vi "main_001.vi"() -> ()   [LabVIEW 2016]
uses:
  ISEGNHQxxu/iseg NHQ VISA Control.ctl
  <vilib>/Analysis/1siggen.llb/Ramp Pattern by Samples.vi
  <vilib>/Utility/file.llb/Read From Spreadsheet File (DBL).vi
  <vilib>/Utility/file.llb/Write Delimited Spreadsheet (string).vi
  <vilib>/Utility/file.llb/Write Delimited Spreadsheet (DBL).vi
  <vilib>/Platform/browser.llb/Open URL in Default Browser (path).vi
  <vilib>/Analysis/NI_AALBase.lvlib
  Newport ESP301/Newport ESP301.lvlib
panel:
  out "noise-o-meter":dbl=nan format="%.1g"
  in  "array size":i32
  out "Waveform Chart":dbl(graph)=159723533.31
  in  "open base path":bool
  in  "Path":path=path "Y:/Ediff/data/2017/01/170106"
  in  "stop":bool
  out "Slide":dbl(slide)=0.99 scale=0.0..1.0
  in  "Tab Control":T1(tab)
  out "esp_pos_fs":dbl caption="[fs]" format="%.6g"
  in  "snap":bool
  in  "dark":bool
  in  "savebin":bool
  in  "savepng":bool
  in  "count?":bool
  in  "dark?":bool
  in  "threshold":i32=110
  in  "t_exp":dbl=0.1 caption="Exposure time [s]"
  in  "dark_load":bool
  in  "frames":i32=100
  in  "avg[t] acc[f]":bool=TRUE
  out "Actual Voltage":dbl[unit]=-0.6 format="%.2f"
  in  "volt_set":bool
  in  "Nominal Voltage":sgl=50.0 max=4000 format="%.2f"
  out "[mm]":dbl format="%.6g"
  in  "esp_rel+":bool
  in  "esp_rel-":bool
  in  "esp_abs_go":bool
  in  "esp_rel_delta":dbl=0.1 caption="delta [mm]" min=0.0
  in  "esp_abs_time":dbl caption="[fs]"
  in  "esp_set_t0":bool
  out "t0 @":dbl format="%.6g"
  in  "esp_abs_dest":dbl caption="[mm]"
  in  "Value in":dbl=2.0 caption="binning"
  in  "delayscan_go":bool
  in  "waypoints":string[][](table)=[["-100000", "5000"], ["50000", ""], ["", ""]]
  in  "delayscan_header":string="DelayScan01" caption="header"
  in  "iterations":i32
  out "XY Graph":cluster{"Array":dbl[], dbl[]}(graph)
  in  "delayscan_stop":bool
  out "Slide 2":dbl(slide)=0.999 scale=0.0..1.0
  in  "meas_stop_volt":bool
  in  "meas_start_volt":bool
  in  "head":string="PowerVoltScan1"
  in  "volt_start":dbl format="%0.2f"
  in  "volt_end":dbl=1.0 format="%0.2f"
  in  "volt_samples":i32=128
  in  "move2com":bool
  in  "meas_start_XY":bool
  in  "showcom":bool
  in  "VISA ISEG":refnum<visa-resource-name>="COM6"
  in  "Channel (A)":enum16{"A", "B"}(ring)=enum."B"
  out "error out":errorcluster
  in  "volt_timeout":u32=6000
  in  "volt_threshold":sgl=2.0 max=4000 format="%.2f"
  in  "esp_axis":i32=2 caption="ESP Axis" min=1 max=3
  in  "esp_visa":refnum<visa-resource-name>="COM1" caption="ESP VISA"
  out "esp301":errorcluster={"status"=TRUE, "code"=-1073807346, "source"="VISA Open in Newport ESP301.lvlib:Initialize.vi->main 0.9.vi"}
  out "captured":dbl[][](graph)
  out "live":dbl[][](graph)
  in  "close":bool
  # "%"
  # "camera"
  # "voltage supply"
  # "delay stage"
  # "absolute"
  # "Axis2"
  # "Axis1"
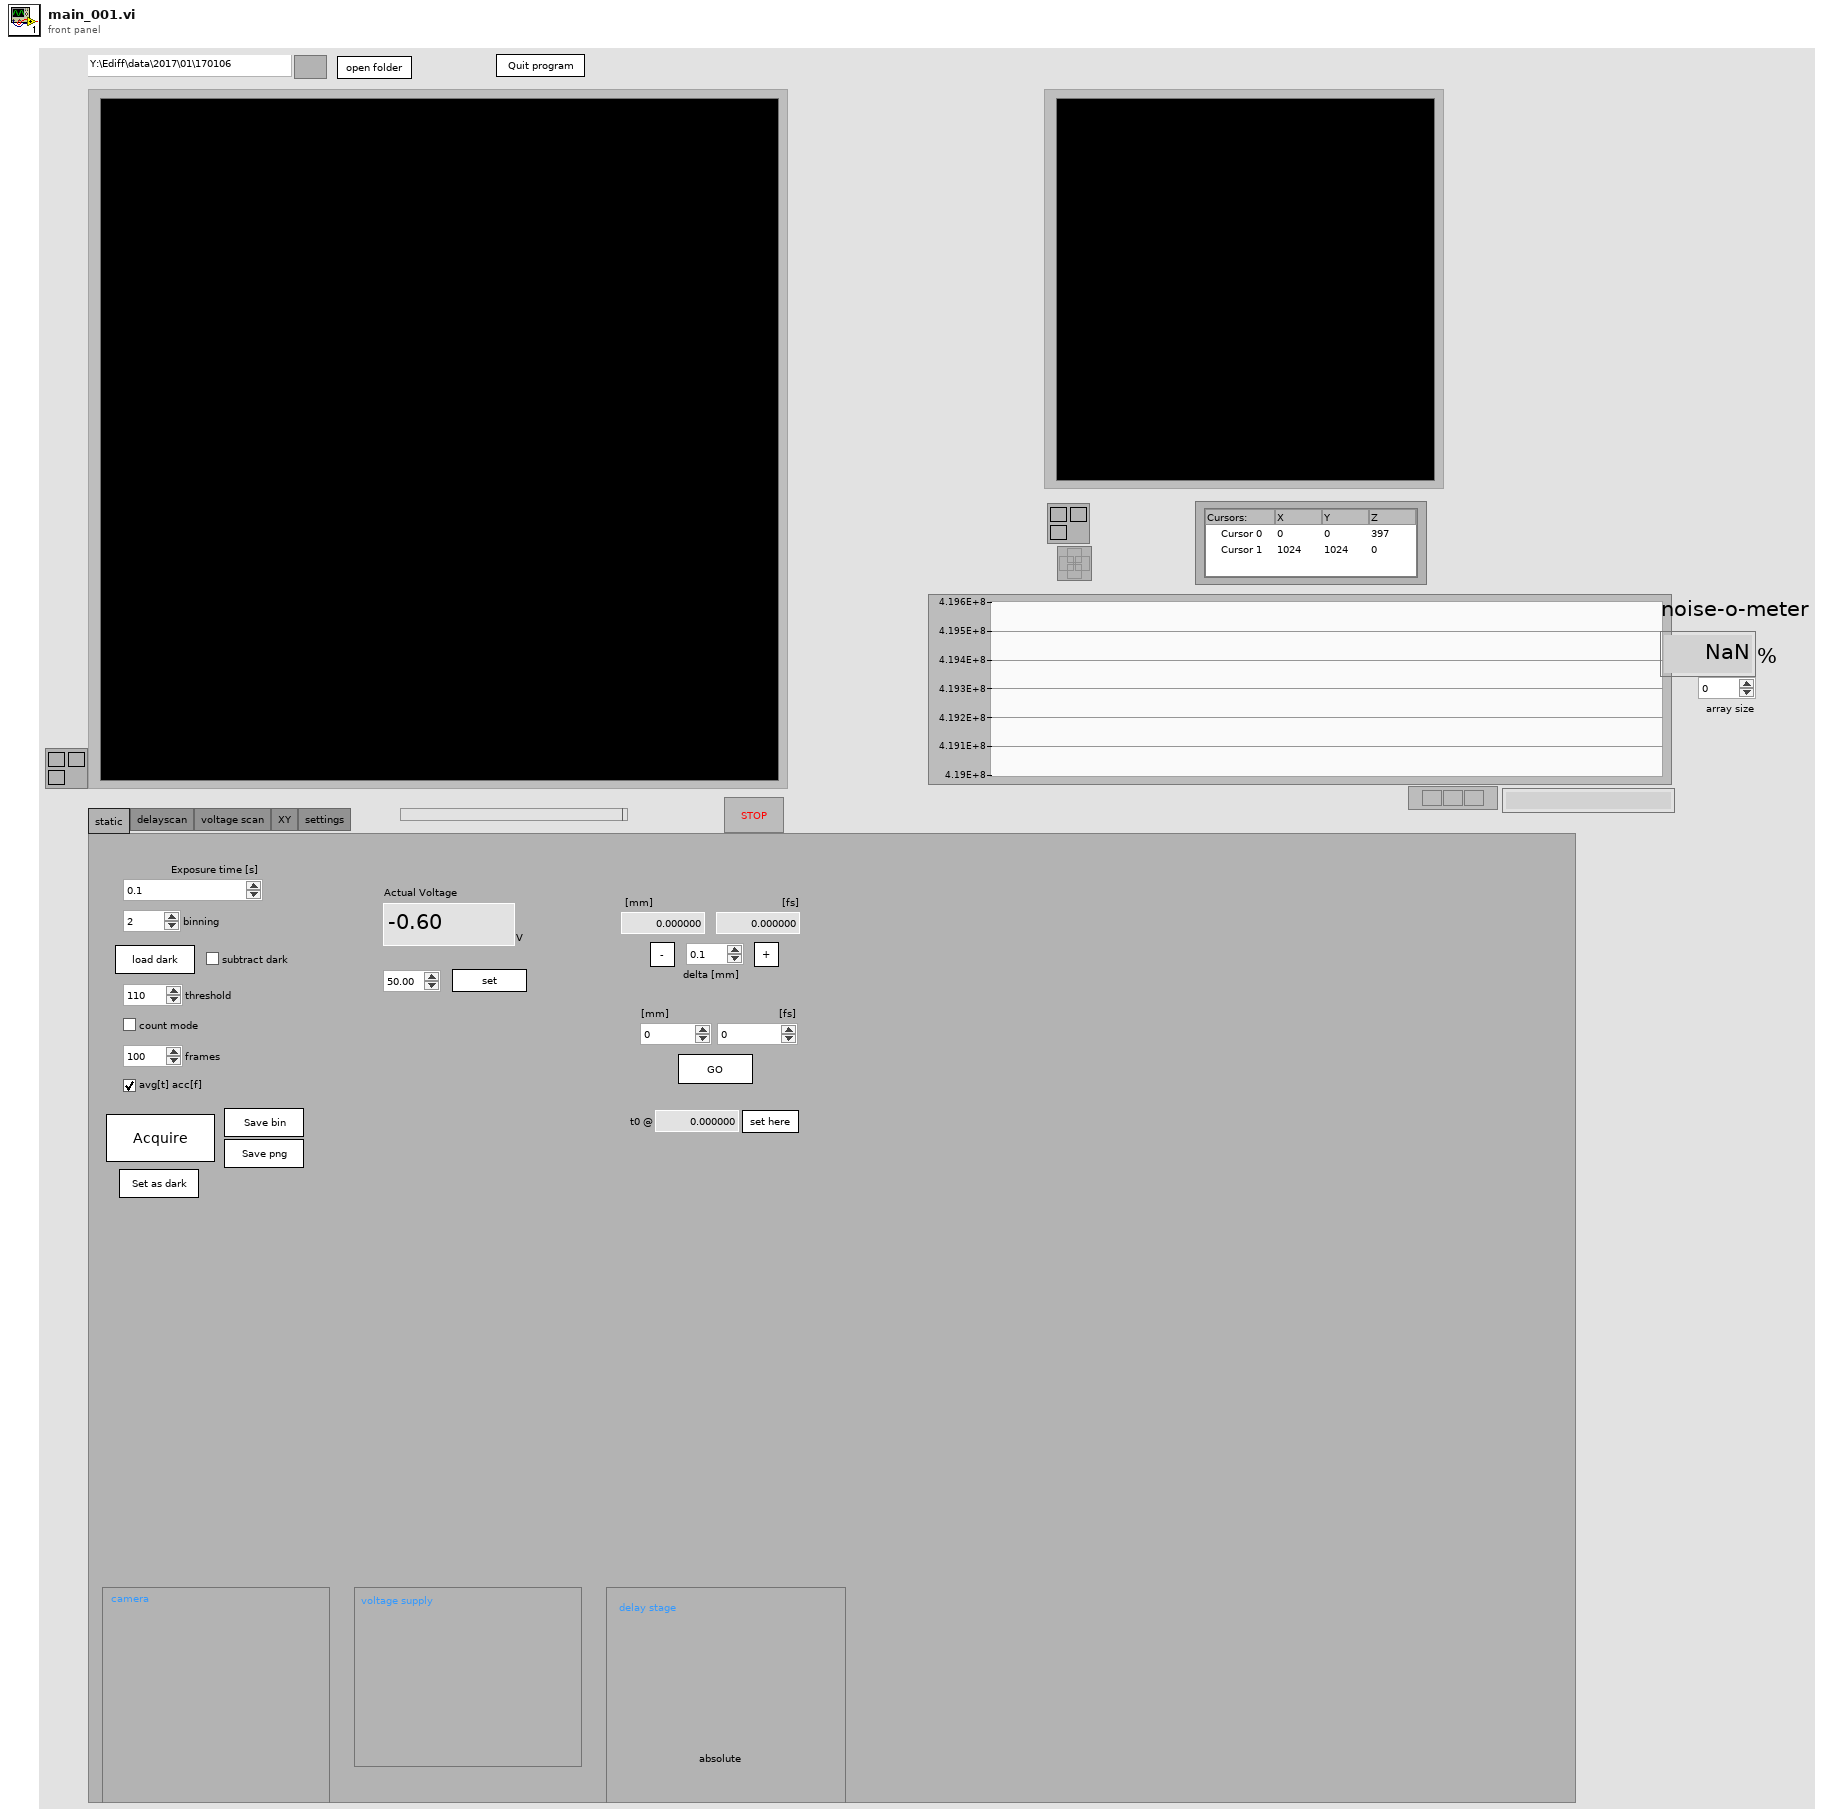
[diagram p1: front panel]
types:
  T1 = enum32{"static", "delayscan", "voltage scan", "XY", "settings"}
  T2 = typedef "Image Type" = u32
  T3 = typedef "IMAQ Image.ctl" = refnum<image>
  T4 = cluster{"height":u32, "width":u32, "datatype":u32}
  T5 = typedef "iseg NHQ VISA Control.ctl" = cluster{"VISA Resource Name":refnum<visa-resource-name>, "FP Notation":bool, "Maximum Voltage":u32, "Maximum Current":u32}
  T6 = cluster{"Axis1 moving":bool, "Axis2 moving":bool, "Axis3 moving":bool, "Axis4 moving":bool, "Motor Power of at least one axis":bool, "Reserved":bool, "Reserved":bool, "Reserved":bool, "Axis5 moving 2":bool, "Axis6 moving 2":bool, "Reserved":bool, "Reserved":bool, "Motor Power of at least one axis":bool, "Reserved":bool, "Reserved":bool, "Reserved":bool}
  T7 = typedef "LVCursorListTypeDef.ctl" = cluster{"Name":string, "Color":u32, "Style":u8, "Point Style":u8, "Name Visible":bool, "Allow Drag":bool, "Cursor Mode":u32, "Plot":i32, "Index":i32, "Position":cluster{"X":dbl, "Y":dbl}, "X Scale":u32, "Y Scale":u32, "Watch Plots":i32[], "Watch All Plots":bool, "Plot Area":i32, "Label Offset":cluster{"X":dbl, "Y":dbl}}[]
  T8 = cluster{"Name":string, "Color":u32, "Style":u8, "Point Style":u8, "Name Visible":bool, "Allow Drag":bool, "Cursor Mode":u32, "Plot":i32, "Index":i32, "Position":cluster{"X":dbl, "Y":dbl}, "X Scale":u32, "Y Scale":u32, "Watch Plots":i32[], "Watch All Plots":bool, "Plot Area":i32, "Label Offset":cluster{"X":dbl, "Y":dbl}}
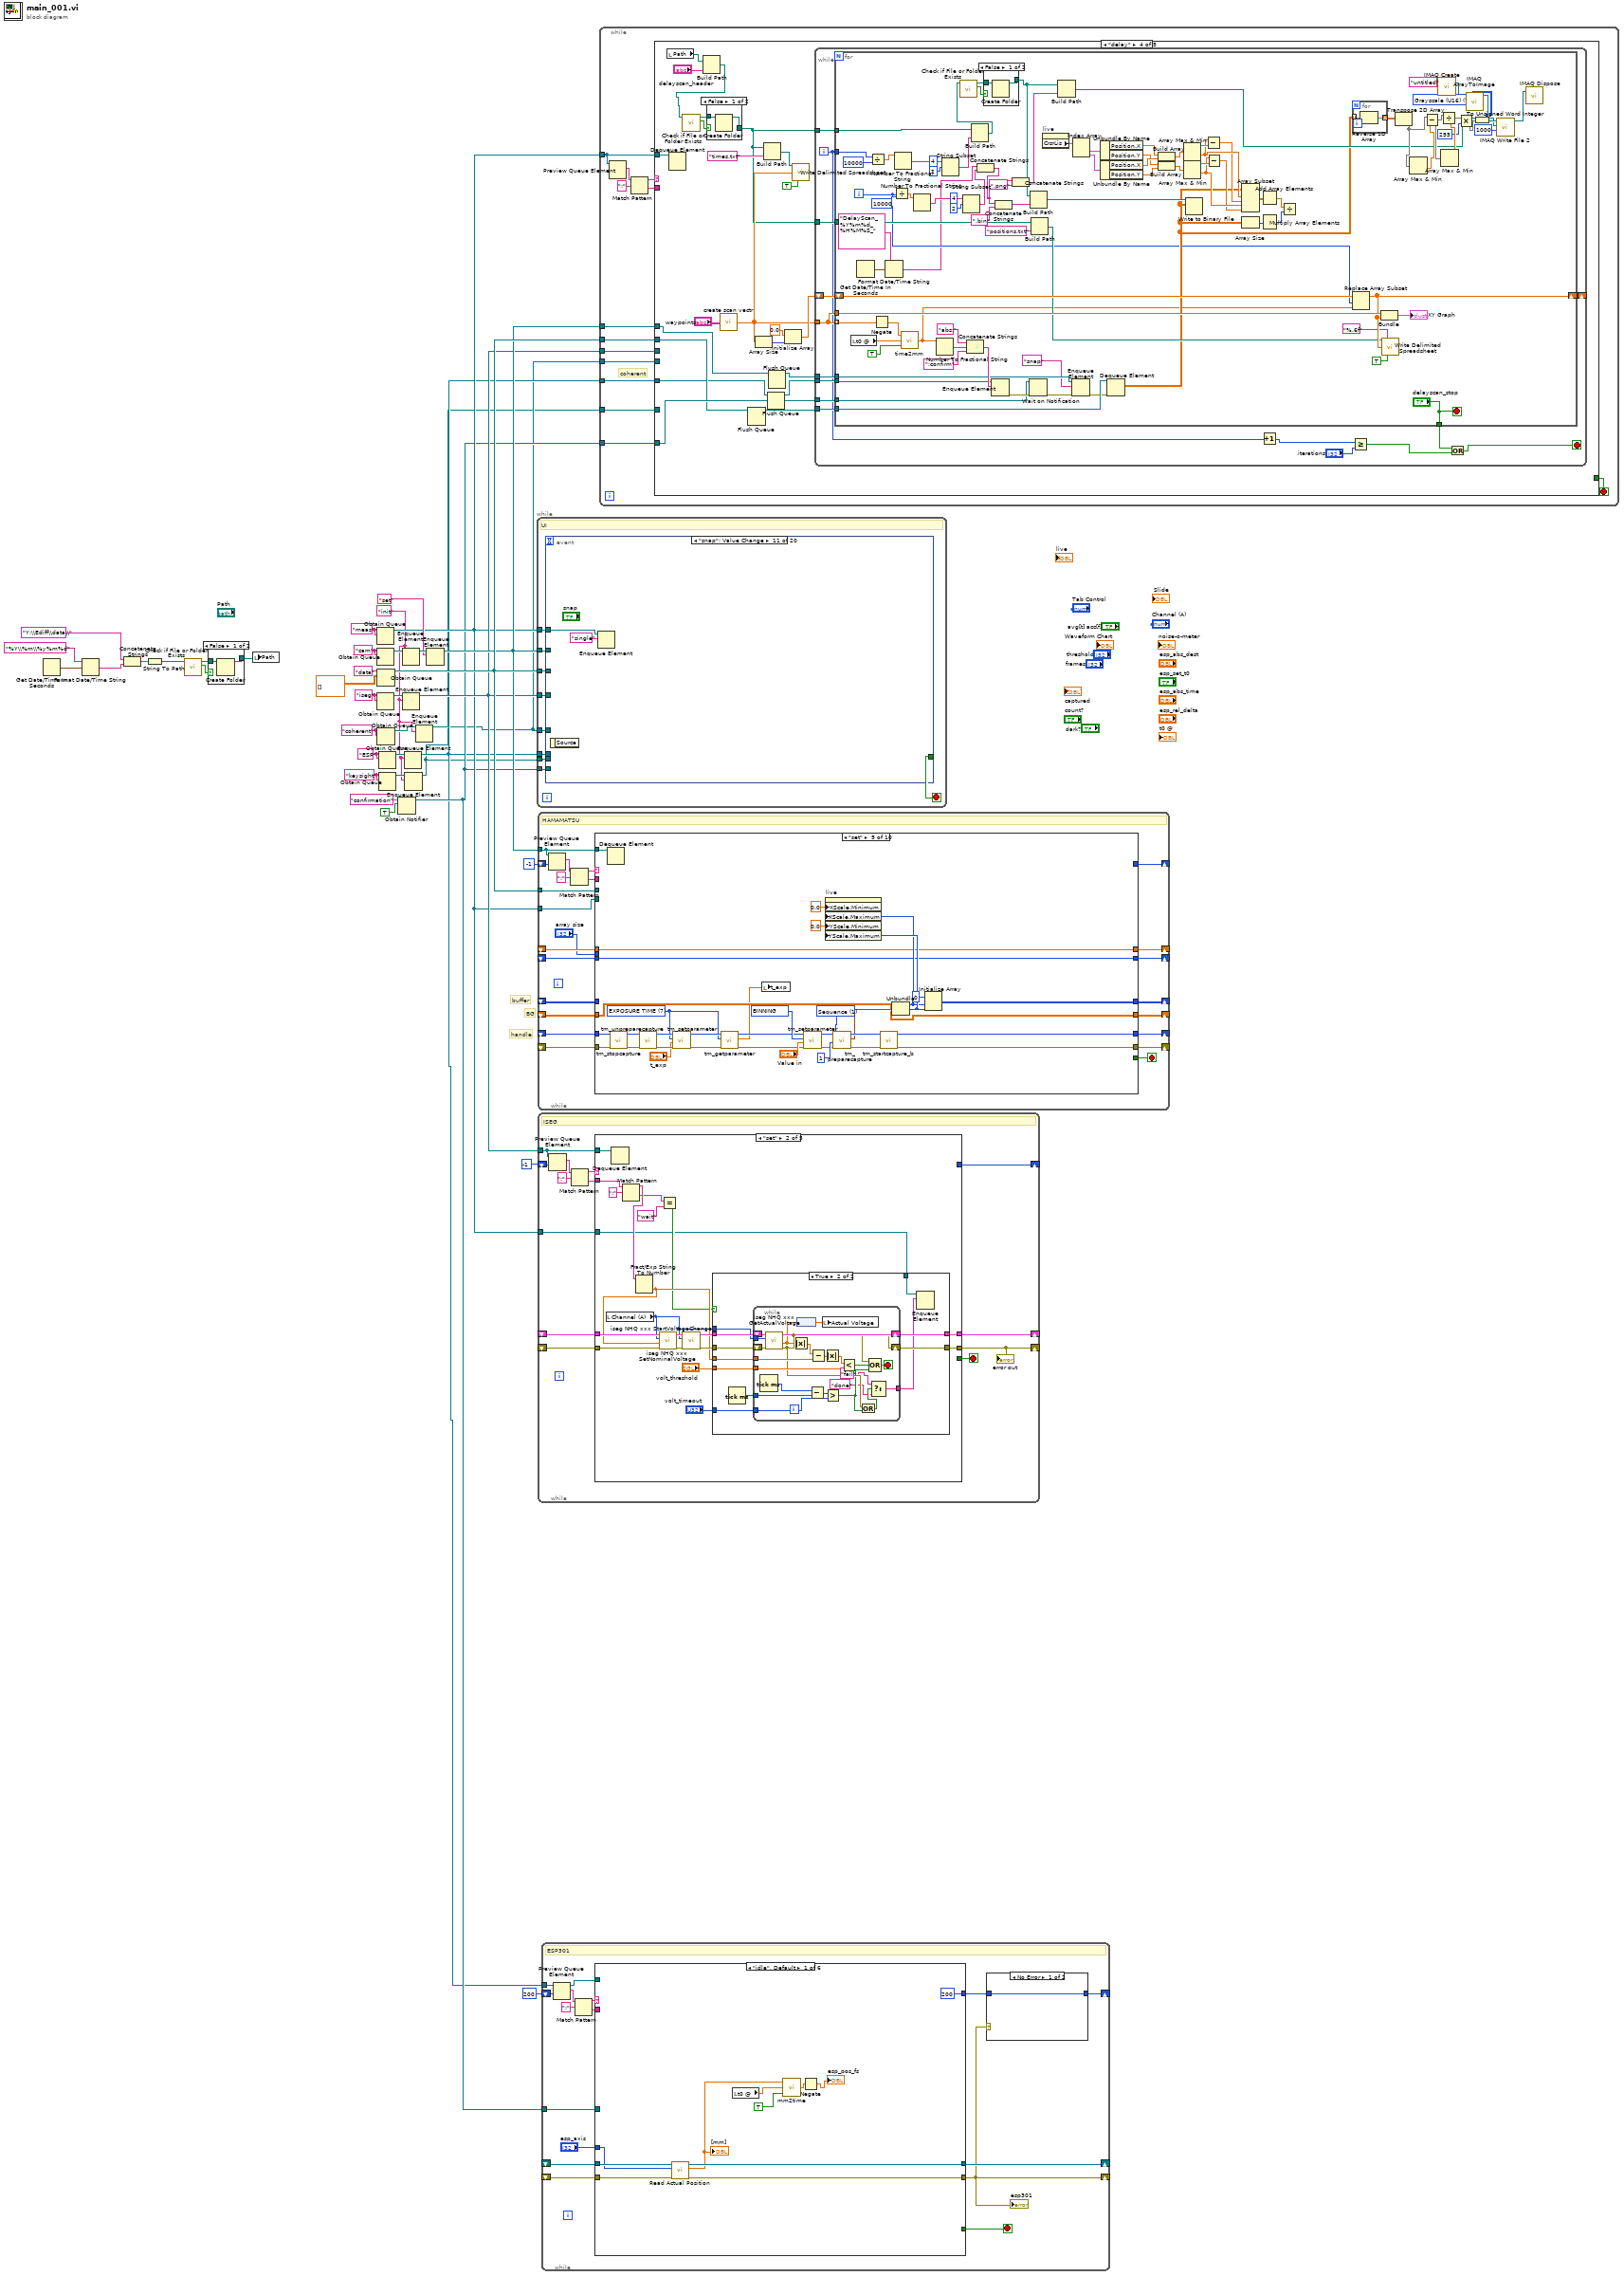
[diagram p0: block diagram]
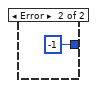
[diagram p3: hidden frame]
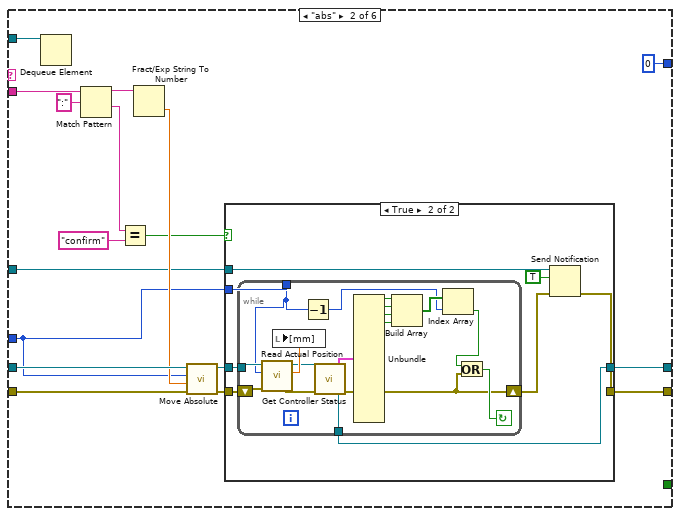
[diagram p4: hidden frame]
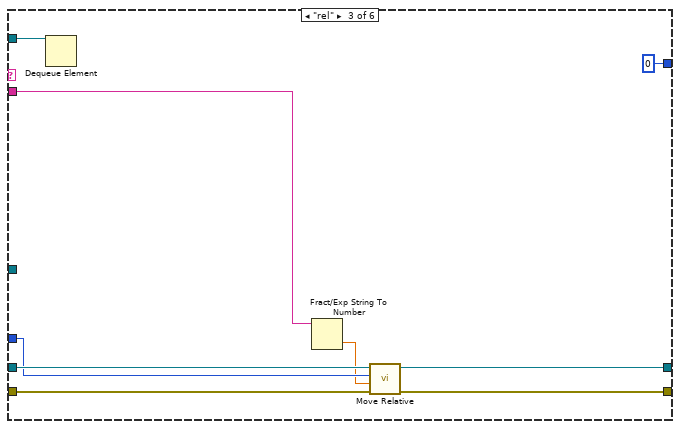
[diagram p6: hidden frame]
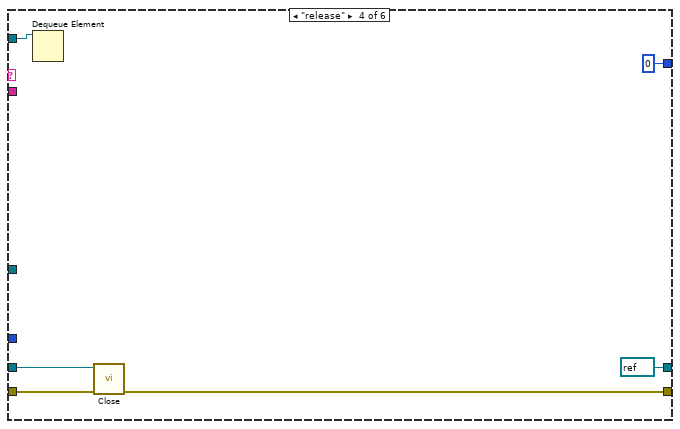
[diagram p7: hidden frame]
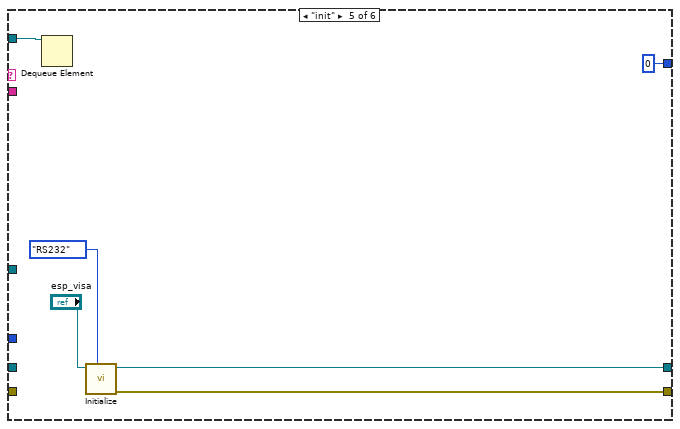
[diagram p8: hidden frame]
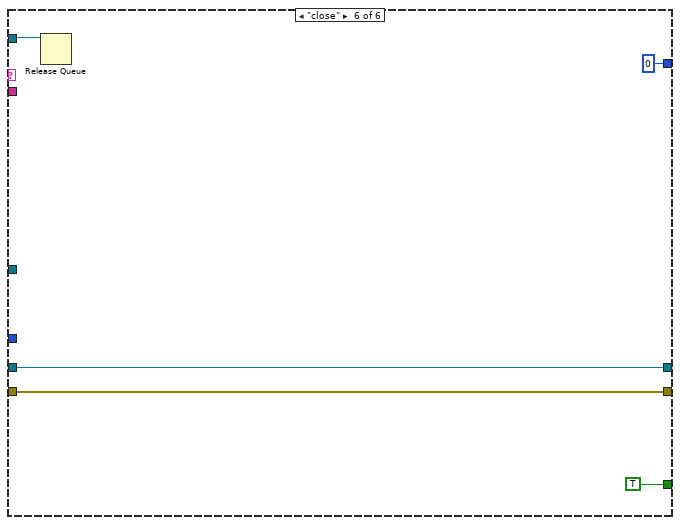
[diagram p9: hidden frame]
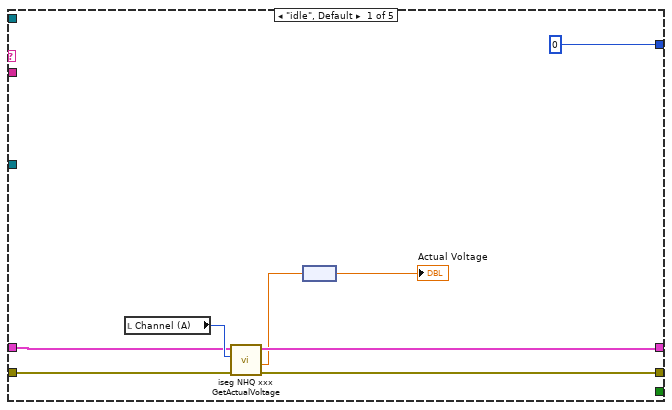
[diagram p10: hidden frame]
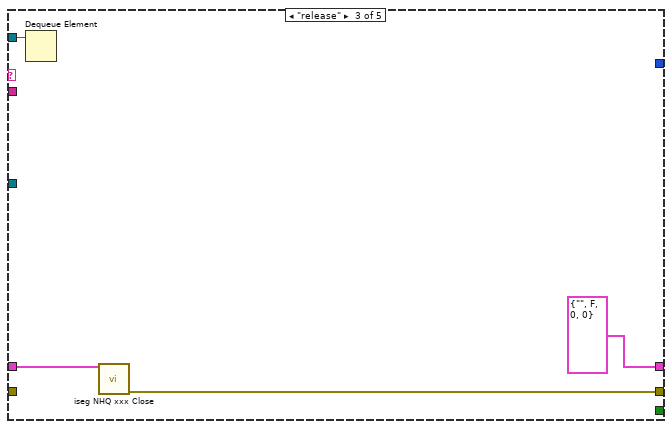
[diagram p12: hidden frame]
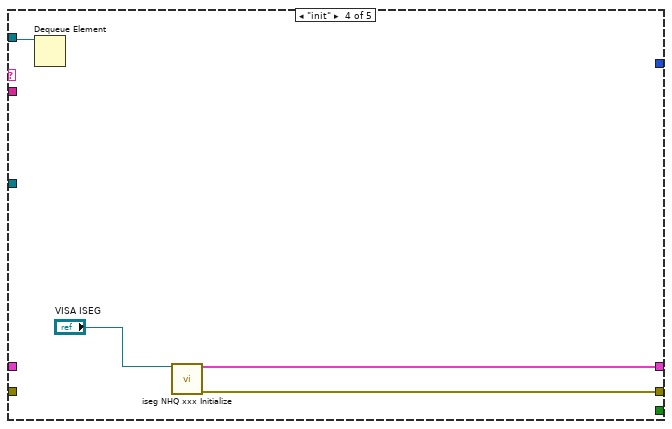
[diagram p13: hidden frame]
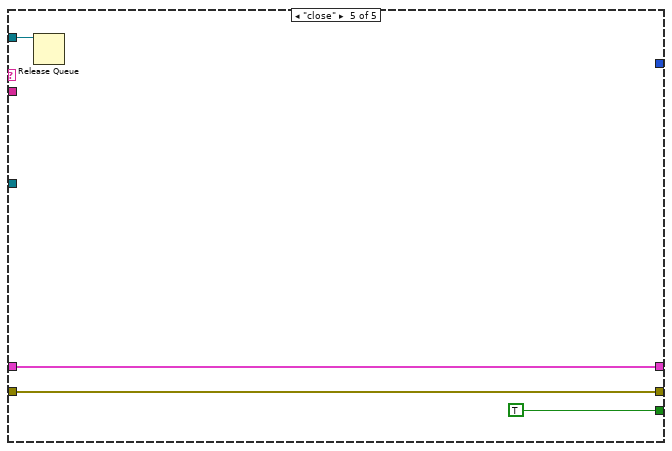
[diagram p14: hidden frame]
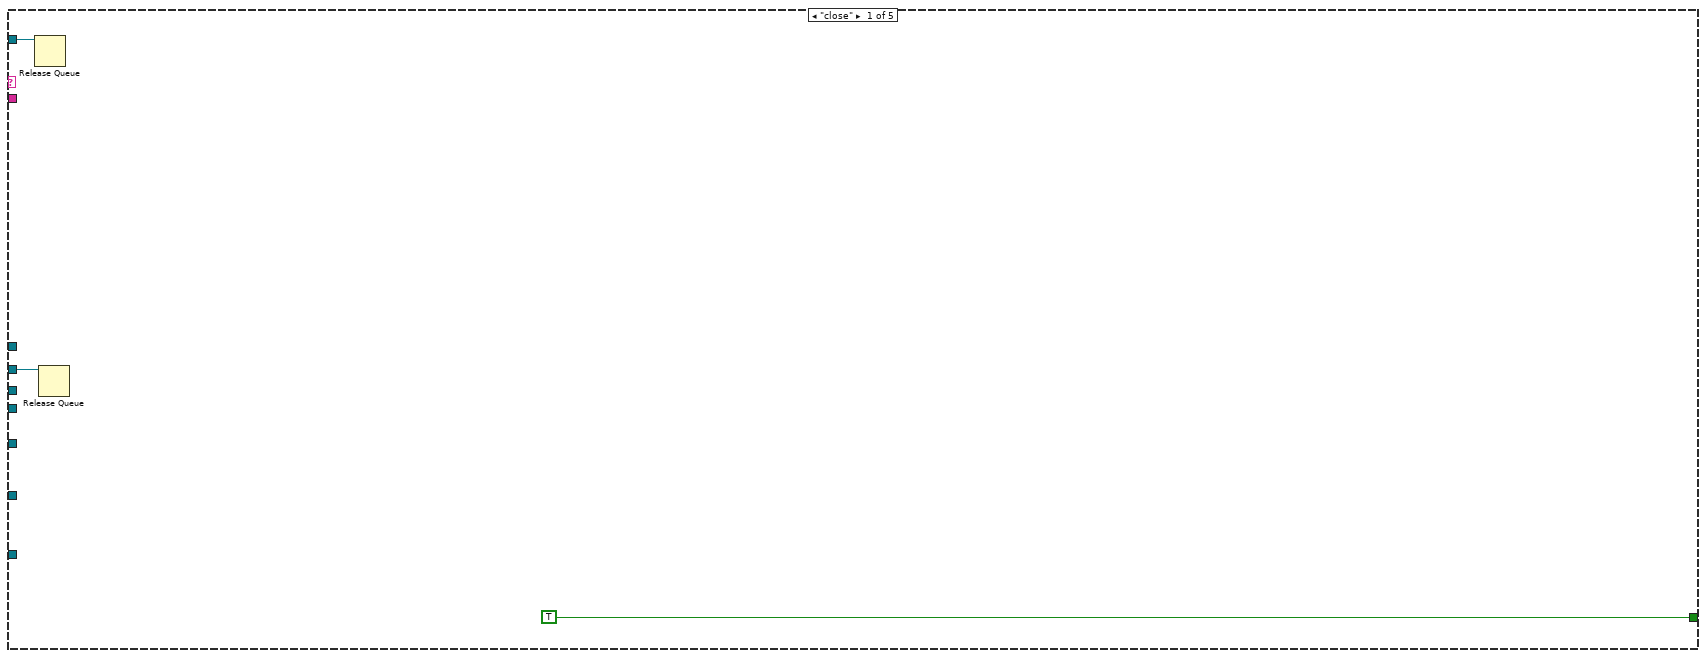
[diagram p15: hidden frame]
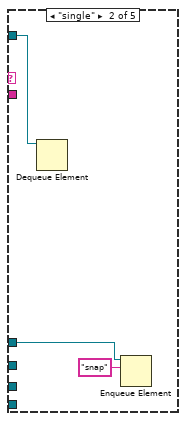
[diagram p16: hidden frame]
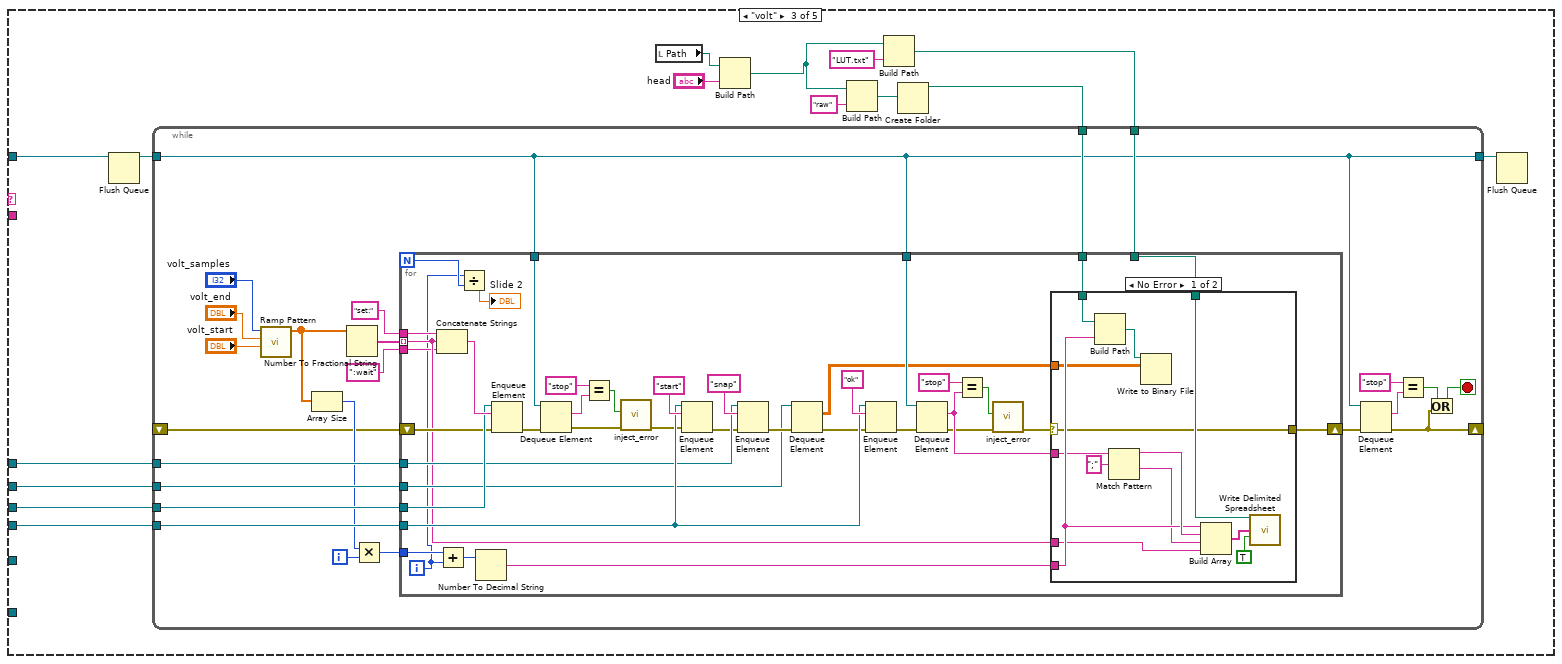
[diagram p17: hidden frame]
diagram:
  w3 = "keysight" ("name (unnamed)")
  w19 = "ESP" ("name (unnamed)")
  w24 = "coherent" ("name (unnamed)")
  w28 = "iseg" ("name (unnamed)")
  w2 = "init" ("element")
  w35 = "meas" ("name (unnamed)")
  w36 = "cam" ("name (unnamed)")
  # "BG"
  # "handle"
  # "buffer"
  n1 = Get Date/Time In Seconds() -> (seconds since 1Jan1904=w16:timestamp)
  n2 = Format Date/Time String(time format string (%c)="%Y\\%m\\%y%m%d", seconds (now)=w16) -> (date/time string=w14:string)  [unwired: 1 in]
  n3 = Concatenate Strings("Y:\\Ediff\\data\\" ("string"), w14) -> (w12:string)
  n4 = String To Path(string=w12) -> (path=w9:path)
  n5 = call <vilib>:"Check if File or Folder Exists.vi"("path"=w9) -> ("file or folder exists?"=w11:bool, "dup path"=w10:path)  [unwired: 8 in, 1 out]
  n6 = case shown="False" w11 {
    tunnel: [w40 w41] -> w8
    tunnel: w10 -> [w39 w41]
    frame False {
      n7 = Create Folder(path (use dialog)=w39) -> (created path=w40:path)  [unwired: 2 in, 2 out]
    }
    frame True {
    }
  }
  n8 = local write "Path"(w8) -> ()
  n9 = Obtain Queue(name (unnamed)=w35, element data type=w35) -> (queue out=w23:refnum<queue>)  [unwired: 3 in, 2 out]
  n10 = Obtain Queue(name (unnamed)=w36, element data type=w36) -> (queue out=w38:refnum<queue>)  [unwired: 3 in, 2 out]
  n11 = Obtain Queue(name (unnamed)=w28, element data type=w28) -> (queue out=w27:refnum<queue>)  [unwired: 3 in, 2 out]
  n12 = Obtain Queue(name (unnamed)="data", element data type=dbl[][] []) -> (queue out=w31:refnum<queue>)  [unwired: 3 in, 2 out]
  n13 = Obtain Queue(name (unnamed)=w24, element data type=w24) -> (queue out=w7:refnum<queue>)  [unwired: 3 in, 2 out]
  n14 = Obtain Queue(name (unnamed)=w19, element data type=w19) -> (queue out=w18:refnum<queue>)  [unwired: 3 in, 2 out]
  n15 = Obtain Queue(name (unnamed)=w3, element data type=w3) -> (queue out=w4:refnum<queue>)  [unwired: 3 in, 2 out]
  n16 = Obtain Notifier(name (unnamed)="confirmation", notification data type=TRUE) -> (notifier out=w20:refnum<notifier>)  [unwired: 2 in, 2 out]
  n17 = Enqueue Element(queue=w38, element=w2) -> (queue out=w34:refnum<queue>)  [unwired: 2 in, 2 out]
  n18 = Enqueue Element(queue=w27, element=w2) -> (queue out=w25:refnum<queue>)  [unwired: 2 in, 2 out]
  n19 = Enqueue Element(queue=w18, element=w2) -> (queue out=w17:refnum<queue>)  [unwired: 2 in, 2 out]
  n20 = Enqueue Element(queue=w4, element=w2) -> (queue out=w1:refnum<queue>)  [unwired: 2 in, 2 out]
  n21 = Enqueue Element(queue=w7, element=w2) -> (queue out=w6:refnum<queue>)  [unwired: 2 in, 2 out]
  n22 = Enqueue Element(queue=w34, element="set") -> (queue out=w30:refnum<queue>)  [unwired: 2 in, 2 out]
  n23 = while {
    tunnel: w30 -> [w50]
    tunnel: w23 -> [w49]
    tunnel: w31 -> [w48]
    tunnel: w25 -> [w46]
    tunnel: w6 -> [w45]
    tunnel: w20 -> [w44]
    tunnel: w17 -> [w43]
    tunnel: w1 -> [w42]
    stop <- w47 stop-if-true
    # "UI"
    n24 = event shown="[10] \"snap\": Value Change" {
      selector: _ -> [_ _ _ _ _ _ _ _ _ _ _ _ _ _ _ _ _ _ _ _]
      dyn-events: _ -> [_ _ _ _ _ _ _ _ _ _ _ _ _ _ _ _ _ _ _ _]
      timeout: _ -> [_ _ _ _ _ _ _ _ _ _ _ _ _ _ _ _ _ _ _ _]
      tunnel: w50 -> [_ w65 _ _ _ _ _ _ w95 w97 _ _ _ _ _ _ w148 _ _ _]
      tunnel: w49 -> [_ w66 _ _ _ _ w88 _ _ _ w98 w101 w102 _ _ w142 _ w155 w157 _]
      tunnel: w48 -> [_ _ _ _ _ _ _ _ _ _ _ _ _ _ _ _ _ _ _ _]
      tunnel: [_ TRUE _ _ _ _ _ _ _ _ _ _ _ _ _ _ _ _ _ _] -> w47
      tunnel: w46 -> [_ w62 _ _ _ _ _ _ _ _ _ _ _ _ _ _ _ _ _ w162]
      tunnel: w45 -> [_ w59 _ _ _ _ _ _ _ _ _ _ _ _ _ _ _ _ _ _]
      tunnel: w44 -> [_ w56 _ _ _ _ _ _ _ _ _ _ _ _ _ _ _ _ _ _]
      tunnel: w43 -> [_ w58 w72 w77 _ _ _ _ _ _ _ _ _ _ _ _ _ _ _ _]
      tunnel: w42 -> [_ w51 _ _ _ _ _ _ _ _ _ _ _ _ _ _ _ _ _ _]
      event Timeout {
        n25 = event-data() -> ()  [unwired: 1 in, 1 out]
      }
      event "close": Value Change {
        w54 = "close" ("element")
        w55 = "release" ("element")
        n26 = event-data() -> ()  [unwired: 1 in, 1 out]
        n27 = Enqueue Element(queue=w59, element=w55) -> (queue out=w60:refnum<queue>)  [unwired: 2 in, 2 out]
        n28 = Enqueue Element(queue=w58, element=w55) -> (queue out=w57:refnum<queue>)  [unwired: 2 in, 2 out]
        n29 = Enqueue Element(queue=w62, element=w55) -> (queue out=w61:refnum<queue>)  [unwired: 2 in, 2 out]
        n30 = Enqueue Element(queue=w65, element=w55) -> (queue out=w64:refnum<queue>)  [unwired: 2 in, 2 out]
        n31 = Enqueue Element(queue=w66, element=w54) -> ()  [unwired: 2 in, 3 out]
        n32 = Enqueue Element(queue=w64, element=w54) -> ()  [unwired: 2 in, 3 out]
        n33 = Enqueue Element(queue=w61, element=w54) -> ()  [unwired: 2 in, 3 out]
        n34 = Enqueue Element(queue=w60, element=w54) -> ()  [unwired: 2 in, 3 out]
        n35 = Enqueue Element(queue=w57, element=w54) -> ()  [unwired: 2 in, 3 out]
        n36 = Release Notifier(notifier=w56) -> ()  [unwired: 2 in, 3 out]
        n37 = Flush Queue(queue=w51) -> (queue out=w52:refnum<queue>)  [unwired: 1 in, 2 out]
        n38 = Enqueue Element(queue=w52, element=w55) -> (queue out=w53:refnum<queue>)  [unwired: 2 in, 2 out]
        n39 = Enqueue Element(queue=w53, element=w54) -> ()  [unwired: 2 in, 3 out]
      }
      event "esp_abs_go": Value Change {
        n40 = event-data() -> ()  [unwired: 1 in, 1 out]
        n41 = local read "esp_abs_dest"() -> (w68:dbl)
        n42 = Number To Fractional String(number=w68) -> (F-format string=w69:string)  [unwired: 3 in]
        n43 = Concatenate Strings("abs:" ("string"), w69, ":confirm" ("string")) -> (w71:string)
        n44 = Enqueue Element(queue=w72, element=w71) -> ()  [unwired: 2 in, 3 out]
      }
      event "esp_rel+", "esp_rel-": Value Change {
        n45 = event-data() -> ()  [unwired: 1 in, 1 out]
        n46 = local read "esp_rel_delta"() -> (w74:dbl)
        n47 = Negate(x=w74) -> (-x=w75:dbl)
        n48 = Select(t=w75, s="esp_rel-", f=w74) -> (s? t:f=w73:dbl)
        n49 = Number To Fractional String(number=w73) -> (F-format string=w79:string)  [unwired: 3 in]
        n50 = Concatenate Strings("rel:" ("string"), w79) -> (w78:string)
        n51 = Enqueue Element(queue=w77, element=w78) -> ()  [unwired: 2 in, 3 out]
      }
      event "esp_set_t0": Value Change {
        n52 = event-data() -> ()  [unwired: 1 in, 1 out]
        n53 = local read "[mm]"() -> (w81:dbl)
        n54 = local write "t0 @"(w81) -> ()
      }
      event "esp_abs_time": Value Change {
        n55 = event-data() -> ()  [unwired: 1 in, 1 out]
        n56 = local read "esp_abs_time"() -> (w83:dbl)
        n57 = local read "t0 @"() -> (w84:dbl)
        n58 = Negate(x=w83) -> (-x=w82:dbl)
        n59 = call "time2mm.vi"("fs[1]/ps[0]"=TRUE, "Offset (mm)"=w84, "time"=w82) -> ("position (mm)"=w85:dbl)
        n60 = local write "esp_abs_dest"(w85) -> ()
      }
      event "delayscan_go": Value Change {
        n61 = event-data() -> ()  [unwired: 1 in, 1 out]
        n62 = Enqueue Element(queue=w88, element="delay") -> ()  [unwired: 2 in, 3 out]
      }
      event "esp_abs_dest": Value Change {
        n63 = event-data() -> ()  [unwired: 1 in, 1 out]
        n64 = local read "esp_abs_dest"() -> (w93:dbl)
        n65 = local read "t0 @"() -> (w92:dbl)
        n66 = call "mm2time.vi"("fs?"=TRUE, "Offset (mm)"=w92, "distance (mm)"=w93) -> ("time in fs/ps seconds"=w90:dbl)
        n67 = Negate(x=w90) -> (-x=w89:dbl)
        n68 = local write "esp_abs_time"(w89) -> ()
      }
      event "dark": Value Change {
        n69 = event-data() -> ()  [unwired: 1 in, 1 out]
        n70 = Enqueue Element(queue=w95, element="dark") -> ()  [unwired: 2 in, 3 out]
      }
      event "t_exp": Value Change {
        n71 = event-data() -> ()  [unwired: 1 in, 1 out]
        n72 = Enqueue Element(queue=w97, element="set") -> ()  [unwired: 2 in, 3 out]
      }
      event "snap": Value Change {
        n73 = event-data() -> ()  [unwired: 1 in, 1 out]
        n74 = Enqueue Element(queue=w98, element="single") -> ()  [unwired: 2 in, 3 out]
      }
      event "meas_start_volt": Value Change {
        n75 = event-data() -> ()  [unwired: 1 in, 1 out]
        n76 = Enqueue Element(queue=w101, element="volt") -> ()  [unwired: 2 in, 3 out]
      }
      event "meas_stop_volt": Value Change {
        n77 = event-data() -> ()  [unwired: 1 in, 1 out]
        n78 = Enqueue Element(queue=w102, element="stop") -> ()  [unwired: 2 in, 3 out]
      }
      event "open base path": Value Change {
        n79 = event-data() -> ()  [unwired: 1 in, 1 out]
        n80 = local read "Path"() -> (w104:path)
        n81 = call-poly <vilib>:"Open URL in Default Browser.vi"("path"=w104) -> ()  [unwired: 5 in, 2 out]
      }
      event "savebin", "savepng": Value Change {
        n82 = event-data() -> ()  [unwired: 1 in, 1 out]
        n83 = Get Date/Time In Seconds() -> (seconds since 1Jan1904=w110:timestamp)
        n84 = local read "Path"() -> (w106:path)
        n85 = Format Date/Time String(time format string (%c)="MCPIMG_%Y%m%d_%H%M%S", seconds (now)=w110) -> (date/time string=w105:string)  [unwired: 1 in]
        n86 = local read "captured"() -> (w107:dbl[][])
        n87 = case shown="False" "savebin" {
          tunnel: w107 -> [w125 w141]
          tunnel: w106 -> [w122 w135]
          tunnel: w105 -> [w120 w136]
          frame False {
            w130 = T2 7 items=["Grayscale (U8)", "Grayscale (I16)", "Grayscale (SGL)", "Complex (CSG)", "RGB (U32)", "HSL (U32)", "RGB (U64)", "Grayscale (U16)"] ("Image Type")
            n88 = for {
              tunnel: w125 -> [w133] mode=indexing
              tunnel: [w132] -> w124 mode=indexing
              n89 = Reverse 1D Array(array=w133) -> (reversed array=w132:dbl[])
            }
            n90 = Concatenate Strings(w120, ".png" ("string")) -> (w121:string)
            n91 = Transpose 2D Array(2D array=w124) -> (transposed array=w113:dbl[][])
            n92 = Array Max & Min(array=w113) -> (min value=w112:dbl)  [unwired: 3 out]
            n93 = Build Path(base path=w122, name or relative path=w121) -> (appended path=w123:path)
            n94 = Subtract(x=w113, y=w112) -> (x-y=w111:dbl[][])
            n95 = call "IMAQ Create"("Image Name"="untitled", "Image Type"=w130) -> ("New Image"=w131:T3)  [unwired: 3 in, 1 out]
            n96 = Array Max & Min(array=w111) -> (max value=w118:dbl)  [unwired: 3 out]
            n97 = Divide(x=w111, y=w118) -> (x/y=w117:dbl[][])
            n98 = Multiply(x=w117, y=255) -> (x*y=w115:dbl[][])
            n99 = To Unsigned Word Integer(number=w115) -> (unsigned 16bit integer=w114:u16[][])
            n100 = call "IMAQ ArrayToImage"("Image Pixels (U16)"=w114, "Image"=w131) -> ("Image Out"=w129:T3)  [unwired: 8 in, 1 out]
            n101 = call-poly "IMAQ Write File 2"("Image Quality"=u32 1000, "File Path"=w123, "Image"=w129) -> ("Image Out (duplicate)"=w127:T3)  [unwired: 7 in, 1 out]
            n102 = call "IMAQ Dispose"("Image"=w127) -> ()  [unwired: 5 in, 1 out]
          }
          frame True {
            n103 = Concatenate Strings(w136, ".bin" ("string")) -> (w138:string)
            n104 = Build Path(base path=w135, name or relative path=w138) -> (appended path=w134:path)
            n105 = Write to Binary File(file (use dialog)=w134, data=w141) -> (refnum out=w140:refnum<file>, error out=w139:errorcluster)  [unwired: 4 in, 1 out]
            n106 = Close File(refnum=w140, error in=w139) -> ()  [unwired: 2 out]
          }
        }
      }
      event "meas_start_XY": Value Change {
        n107 = event-data() -> ()  [unwired: 1 in, 1 out]
        n108 = Enqueue Element(queue=w142, element="XY") -> ()  [unwired: 2 in, 3 out]
      }
      event "dark_load": Value Change {
        n109 = event-data() -> ()  [unwired: 1 in, 1 out]
        n110 = local read "Path"() -> (w147:path)
        n111 = call "File Dialog"("start path"=w147) -> ("selected path"=w145:path, "cancelled"=w144:bool)  [unwired: 11 in, 2 out]
        n112 = case shown="False" w144 {
          tunnel: w148 -> [w153 _]
          tunnel: "dark_load:" ("element") -> [w151 _]
          tunnel: w145 -> [w149 _]
          frame False {
            n113 = Path To String(path=w149) -> (string=w150:string)
            n114 = Concatenate Strings(w151, w150) -> (w152:string)
            n115 = Enqueue Element(queue=w153, element=w152) -> ()  [unwired: 2 in, 3 out]
          }
          frame True {
          }
        }
      }
      event "move2com": Value Change {
        n116 = event-data() -> ()  [unwired: 1 in, 1 out]
        n117 = Enqueue Element(queue=w155, element="mov2cursor") -> ()  [unwired: 2 in, 3 out]
      }
      event "showcom": Value Change {
        n118 = event-data() -> ()  [unwired: 1 in, 1 out]
        n119 = Enqueue Element(queue=w157, element="showcom") -> ()  [unwired: 2 in, 3 out]
      }
      event "volt_set": Value Change {
        n120 = event-data() -> ()  [unwired: 1 in, 1 out]
        n121 = Number To Fractional String(number="Nominal Voltage") -> (F-format string=w158:string)  [unwired: 3 in]
        n122 = Concatenate Strings("set:" ("element"), w158) -> (w161:string)
        n123 = Enqueue Element(queue=w162, element=w161) -> ()  [unwired: 2 in, 3 out]
      }
    }
  }
  n124 = while {
    tunnel: w30 -> [w181]
    shift-right: [w179] -> _
    shift-left: _ -> [w178]
    shift-right: [w177] -> _
    shift-left: _ -> [w176]
    shift-right: [w175] -> _
    shift-left: _ -> [w174]
    shift-right: [w173] -> _
    shift-left: _ -> [w172]
    shift-right: [w170] -> _
    shift-left: -1 -> [w171]
    tunnel: w31 -> [w169]
    tunnel: w23 -> [w168]
    shift-right: [w167] -> _
    shift-left: _ -> [w166]
    shift-right: [w164] -> _
    shift-left: _ -> [w165]
    stop <- w180 stop-if-true
    # "HAMAMATSU"
    n125 = Preview Queue Element(queue=w181, timeout in ms (-1)=w171) -> (element=w185:string)  [unwired: 1 in, 3 out]
    n126 = Match Pattern(string=w185, regular expression=":") -> (before substring=w183:string, after substring=w182:string)  [unwired: 1 in, 2 out]
    n127 = case shown="\"set\"" w183 {
      tunnel: w182 -> [_ _ w285 _ _ w375 _ _ _ _]
      tunnel: w181 -> [_ w224 w286 w320 w369 w379 w391 w394 w420 w442]
      tunnel: [_ _ _ _ _ _ _ _ _ TRUE] -> w180
      tunnel: [w204 w226 w289 w325 w367 w376 w383 w399 w408 w437] -> w179
      tunnel: w178 -> [w206 w229 w291 w327 w367 w376 w387 _ w434 w437]
      tunnel: [w205 w221 w290 w324 w366 w377 u32 0 ("Handle out") w397 w409 w438] -> w177
      tunnel: w176 -> [w207 w227 w292 w328 w366 w377 w388 _ w432 w438]
      tunnel: [w203 w228 w284 w323 w368 w378 w389 w395 w421 w439] -> w175
      tunnel: w174 -> [w203 w228 w284 w323 w368 w378 w389 w395 _ w439]
      tunnel: [w202 w225 w293 w326 w365 w372 w390 w396 w412 w440] -> w173
      tunnel: w172 -> [w202 w225 w293 w326 _ _ w390 w396 w412 w440]
      tunnel: [0 _ _ _ _ _ _ _ _ _] -> w170
      tunnel: w169 -> [_ w220 w294 _ _ _ _ _ _ _]
      tunnel: w168 -> [_ _ _ w321 _ _ _ _ _ _]
      tunnel: [w188 w215 w288 w312 w364 w371 w381 w393 w414 w436] -> w167
      tunnel: w166 -> [w197 w218 w288 w315 w364 w371 w381 w393 w414 w436]
      tunnel: w165 -> [w192 w217 w287 w313 w363 w370 w380 w392 w413 w435]
      tunnel: [w191 w214 w287 w311 w363 w370 w380 w392 w413 w435] -> w164
      tunnel: "array size" -> [w190 w216 _ w314 _ _ _ _ _ _]
      frame "idle", Default {
        n128 = local read "threshold"() -> (w208:i32)
        n129 = call "tm_getnextframe_a.vi"("error in (no error)"=w206, "Buffer"=w203, "Handle in"=w207) -> ("error out"=w204:errorcluster, "Data"=w198:u16[][], "Handle out"=w205:u32)  [unwired: 6 in]
        n130 = local read "dark?"() -> (w209:bool)
        n131 = local read "count?"() -> (w199:bool)
        n132 = case shown="False" w209 {
          tunnel: [w210 w213] -> w200
          tunnel: w198 -> [w210 w212]
          tunnel: w202 -> [_ w211]
          frame False {
          }
          frame True {
            n133 = Subtract(x=w212, y=w211) -> (x-y=w213:dbl[][])
          }
        }
        n134 = call "filtr_b.vi"("count?"=w199, "threshold"=w208, "input array"=w200) -> ("output array"=w186:dbl[][])  [unwired: 8 in]
        n135 = Add Array Elements(numeric array=w186) -> (sum=w187:dbl)
        n136 = call "ringbuffer.vi"("new val"=w187, "index in"=w192, "array size"=w190, "array in"=w197) -> ("index out"=w191:i32, "array out"=w188:dbl[])  [unwired: 6 in]
        n137 = local write "live"(w186) -> ()
        n138 = local write "Waveform Chart"(w187) -> ()
        n139 = call <vilib>:"Std Deviation and Variance.vi"("X"=w188) -> ("mean"=w193:dbl, "standard deviation"=w196:dbl)  [unwired: 1 in, 1 out]
        n140 = Divide(x=w196, y=w193) -> (x/y=w195:dbl)
        n141 = Multiply(x=w195, y=100.0) -> (x*y=w189:dbl)
        n142 = local write "noise-o-meter"(w189) -> ()
      }
      frame "snap" {
        n143 = Dequeue Element(queue=w224) -> ()  [unwired: 2 in, 4 out]
        n144 = local read "avg[t] acc[f]"() -> (w223:bool)
        n145 = local read "threshold"() -> (w231:i32)
        n146 = local read "frames"() -> (w230:i32)
        n147 = local read "count?"() -> (w222:bool)
        n148 = local read "dark?"() -> (w232:bool)
        n149 = for {
          N: w230 -> [w250]
          tunnel: w232 -> [w264]
          tunnel: w228 -> [w262]
          tunnel: w227 -> [w263]
          tunnel: w231 -> [w256]
          tunnel: [w260] -> w221
          shift-right: [w259] -> w226
          shift-left: w229 -> [w261]
          tunnel: w225 -> [w255]
          shift-right: [w233] -> w219
          shift-left: w228 -> [w253]
          tunnel: w223 -> [w254]
          tunnel: w222 -> [w252]
          shift-right: [w243] -> w215
          shift-left: w218 -> [w244]
          tunnel: w216 -> [w241]
          shift-right: [w240] -> w214
          shift-left: w217 -> [w242]
          shift-right: [w236] -> _
          shift-left: _ -> [w237]
          i -> [w251]
          stop <- "stop" stop-if-true
          n150 = call "tm_getnextframe_a.vi"("error in (no error)"=w261, "Buffer"=w262, "Handle in"=w263) -> ("error out"=w259:errorcluster, "Data"=w258:u16[][], "Handle out"=w260:u32)  [unwired: 6 in]
          n151 = Divide(x=w251, y=w250) -> (x/y=w249:dbl)
          n152 = case shown="True" w264 {
            tunnel: [w275 w278] -> w257
            tunnel: w258 -> [w275 w277]
            tunnel: w255 -> [_ w276]
            frame False {
            }
            frame True {
              n153 = Subtract(x=w277, y=w276) -> (x-y=w278:dbl[][])
            }
          }
          n154 = local write "Slide"(w249) -> ()
          n155 = Tick Count (ms)() -> (millisecond timer value=w236:u32)
          n156 = call "filtr_b.vi"("count?"=w252, "threshold"=w256, "input array"=w257) -> ("output array"=w235:dbl[][])  [unwired: 8 in]
          n157 = Subtract(x=w236, y=w237) -> ()  [unwired: 1 out]
          n158 = Add Array Elements(numeric array=w235) -> (sum=w234:dbl)
          n159 = call "ringbuffer.vi"("new val"=w234, "index in"=w242, "array size"=w241, "array in"=w244) -> ("index out"=w240:i32, "array out"=w243:dbl[])  [unwired: 6 in]
          n160 = call <vilib>:"Std Deviation and Variance.vi"("X"=w243) -> ("mean"=w245:dbl, "standard deviation"=w247:dbl)  [unwired: 1 in, 1 out]
          n161 = local write "live"(w235) -> ()
          n162 = local write "Waveform Chart"(w234) -> ()
          n163 = Divide(x=w247, y=w245) -> (x/y=w239:dbl)
          n164 = case shown="True" w254 {
            tunnel: w253 -> [w267 w274]
            tunnel: w235 -> [w266 w272]
            tunnel: [w265 w268] -> w233
            tunnel: w251 -> [_ w269]
            frame False {
              n165 = Add(x=w267, y=w266) -> (x+y=w265:dbl[][])
            }
            frame True {
              n166 = Multiply(x=w274, y=w269) -> (x*y=w273:dbl[][])
              n167 = Increment(x=w269) -> (x+1=w270:i32)
              n168 = Add(x=w273, y=w272) -> (x+y=w271:dbl[][])
              n169 = Divide(x=w271, y=w270) -> (x/y=w268:dbl[][])
            }
          }
          n170 = local write "captured"(w233) -> ()
          n171 = Multiply(x=w239, y=100.0) -> (x*y=w238:dbl)
          n172 = local write "noise-o-meter"(w238) -> ()
        }
        n173 = local write "captured"(w219) -> ()
        n174 = Enqueue Element(queue=w220, element=w219) -> ()  [unwired: 2 in, 3 out]
      }
      frame "single" {
        n175 = Dequeue Element(queue=w286) -> ()  [unwired: 2 in, 4 out]
        n176 = Decimal String To Number(string=w285) -> (number=w280:i32)  [unwired: 2 in, 1 out]
        n177 = To Unsigned Quad Integer(1:w284) -> (0:w283:u64[][])
        n178 = for {
          N: w280 -> [_]
          tunnel: w284 -> [w306]
          tunnel: w292 -> [w305]
          tunnel: w291 -> [w304]
          tunnel: [w303] -> w290
          tunnel: [w302] -> w289
          shift-right: [w299] -> w282
          shift-left: w283 -> [w301]
          n179 = call "tm_getnextframe_a.vi"("error in (no error)"=w304, "Buffer"=w306, "Handle in"=w305) -> ("error out"=w302:errorcluster, "Data"=w300:u16[][], "Handle out"=w303:u32)  [unwired: 6 in]
          n180 = Add(x=w300, y=w301) -> (x+y=w299:u64[][])
        }
        n181 = local read "dark?"() -> (w295:bool)
        n182 = Divide(x=w282, y=w280) -> (x/y=w281:dbl[][])
        n183 = case shown="True" w295 {
          tunnel: [w307 w310] -> w298
          tunnel: w281 -> [w307 w309]
          tunnel: w293 -> [_ w308]
          frame False {
          }
          frame True {
            n184 = Subtract(x=w309, y=w308) -> (x-y=w310:dbl[][])
          }
        }
        n185 = local read "threshold"() -> (w296:i32)
        n186 = local read "count?"() -> (w297:bool)
        n187 = call "filtr_b.vi"("count?"=w297, "threshold"=w296, "input array"=w298) -> ("output array"=w279:dbl[][])  [unwired: 8 in]
        n188 = Enqueue Element(queue=w294, element=w279) -> ()  [unwired: 2 in, 3 out]
        n189 = local write "captured"(w279) -> ()
      }
      frame "snap_I" {
        n190 = Dequeue Element(queue=w320) -> ()  [unwired: 2 in, 4 out]
        n191 = local read "threshold"() -> (w331:i32)
        n192 = local read "frames"() -> (w330:i32)
        n193 = local read "count?"() -> (w329:bool)
        n194 = local read "dark?"() -> (w332:bool)
        n195 = for {
          N: w330 -> [w346]
          tunnel: w332 -> [w358]
          tunnel: w323 -> [w356]
          tunnel: w328 -> [w357]
          tunnel: w331 -> [w350]
          tunnel: [w354] -> w324
          shift-right: [w353] -> w325
          shift-left: w327 -> [w355]
          tunnel: w326 -> [w349]
          tunnel: w329 -> [w348]
          tunnel: [w344] -> w322 mode=indexing
          shift-right: [w336] -> w312
          shift-left: w315 -> [w337]
          tunnel: w314 -> [w335]
          shift-right: [w333] -> w311
          shift-left: w313 -> [w334]
          i -> [w347]
          n196 = call "tm_getnextframe_a.vi"("error in (no error)"=w355, "Buffer"=w356, "Handle in"=w357) -> ("error out"=w353:errorcluster, "Data"=w352:u16[][], "Handle out"=w354:u32)  [unwired: 6 in]
          n197 = call "ringbuffer.vi"("index in"=w334, "array size"=w335, "array in"=w337) -> ("index out"=w333:i32, "array out"=w336:dbl[])  [unwired: 7 in]
          n198 = Divide(x=w347, y=w346) -> (x/y=w345:dbl)
          n199 = case shown="True" w358 {
            tunnel: [w359 w362] -> w351
            tunnel: w352 -> [w359 w361]
            tunnel: w349 -> [_ w360]
            frame False {
            }
            frame True {
              n200 = Subtract(x=w361, y=w360) -> (x-y=w362:dbl[][])
            }
          }
          n201 = local write "Slide"(w345) -> ()
          n202 = call <vilib>:"Std Deviation and Variance.vi"("X"=w336) -> ("mean"=w338:dbl, "standard deviation"=w341:dbl)  [unwired: 1 in, 1 out]
          n203 = call "filtr_b.vi"("count?"=w348, "threshold"=w350, "input array"=w351) -> ("output array"=w343:dbl[][])  [unwired: 8 in]
          n204 = Divide(x=w341, y=w338) -> (x/y=w340:dbl)
          n205 = local write "live"(w343) -> ()
          n206 = Multiply(x=w340, y=100.0) -> (x*y=w342:dbl)
          n207 = local write "noise-o-meter"(w342) -> ()
          n208 = Add Array Elements(numeric array=w343) -> (sum=w344:dbl)
          n209 = local write "Waveform Chart"(w344) -> ()
        }
        n210 = call <vilib>:"Std Deviation and Variance.vi"("X"=w322) -> ("mean"=w319:dbl, "standard deviation"=w318:dbl)  [unwired: 1 in, 1 out]
        n211 = Format Into String(format string="%.6e;%.6e", w319, w318) -> (resulting string=w317:string)  [unwired: 2 in, 1 out]
        n212 = Enqueue Element(queue=w321, element=w317) -> ()  [unwired: 2 in, 3 out]
      }
      frame "dark" {
        n213 = Dequeue Element(queue=w369) -> ()  [unwired: 2 in, 4 out]
        n214 = local read "captured"() -> (w365:dbl[][])
      }
      frame "dark_load" {
        n215 = Dequeue Element(queue=w379) -> ()  [unwired: 2 in, 4 out]
        n216 = String To Path(string=w375) -> (path=w374:path)
        n217 = Read from Binary File(5:dbl[][] [] ("all rows"), 11:w374) -> (2:w372:dbl[][])  [unwired: 4 in, 3 out]
        n218 = call-poly <vilib>:"Read From Spreadsheet File.vi"("file path (dialog if empty)"=w374) -> ()  [unwired: 6 in, 5 out]
      }
      frame "release" {
        n219 = call "tm_stopcapture.vi"("error in (no error)"=w387, "Handle in"=w388) -> ("error out"=w385:errorcluster, "Handle out"=w386:u32)  [unwired: 8 in]
        n220 = Dequeue Element(queue=w391) -> ()  [unwired: 2 in, 4 out]
        n221 = call "tm_closecamera.vi"("error in (no error)"=w385, "Handle in"=w386) -> ("error out"=w384:errorcluster)  [unwired: 9 in]
        n222 = call "tm_deinitialize.vi"("error in (no error)"=w384) -> ("error out"=w383:errorcluster)  [unwired: 10 in]
      }
      frame "init" {
        n223 = Dequeue Element(queue=w394) -> ()  [unwired: 2 in, 4 out]
        n224 = call "tm_initialize.vi"() -> ("error out"=w400:errorcluster)  [unwired: 8 in, 3 out]
        n225 = call "tm_opencamera.vi"("error in (no error)"=w400, "Camera Index"=u32 0) -> ("error out"=w399:errorcluster, "Handle out"=w397:u32)  [unwired: 7 in, 1 out]
      }
      frame "set" {
        w426 = 1 items=["Snap", "Sequence"] ("Capture mode")
        w427 = u32 4215968 items=["BINNING"=4215968, "BITS PER CHANNEL"=2, "ACTIVE VIEW INDEX"=3, "CCD MODE"=4, "SENSOR MODE"=5, "READOUT MODE"=6, "EXPOSURE TIME"=7, "CONTRAST GAIN"=8, "CONTRAST OFFSET"=9, "LIGHT MODE"=10, "SENSITIVITY"=11, "WHITE BALANCE"=12, "PHOTON IMAGING MODE"=13, "HIGH DYNAMIC RANGE MODE"=14, "TRIGGER SOURCE"=15, "TRIGGER ACTIVE"=16, "TRIGGER MODE"=17, "TRIGGER POLARITY"=18, "TRIGGER GLOBAL EXPOSURE"=19, "FIRST TRIGGER BEHAVIOR"=20, "TRIGGER TIMES"=21, "OUTPUT TRIGGER POLARITY"=22, "OUTPUT TRIGGER DELAY"=23, "OUTPUT TRIGGER PERIOD"=24, "TEMPERATURE"=25, "TEMPERATURE TARGET"=26, "SENSOR COOLER FAN"=27, "MECHANICAL SHUTTER"=28, "BACK FOCUS POSITION"=29, "FRAMEBUNDLE MODE"=30, "FRAMEBUNDLE NUMBER"=31, "LINEBUNDLE HEIGHT"=32, "TRIGGER CONNECTOR"=33, "IMAGE PIXEL TYPE"=34, "OUTPUT TRIGGER KIND"=35, "READOUT DIRECTION"=36, "CHANNEL SYNC"=37] ("Parameter")
        w404 = u32 7 items=["BINNING"=4215968, "BITS PER CHANNEL"=2, "ACTIVE VIEW INDEX"=3, "CCD MODE"=4, "SENSOR MODE"=5, "READOUT MODE"=6, "EXPOSURE TIME"=7, "CONTRAST GAIN"=8, "CONTRAST OFFSET"=9, "LIGHT MODE"=10, "SENSITIVITY"=11, "WHITE BALANCE"=12, "PHOTON IMAGING MODE"=13, "HIGH DYNAMIC RANGE MODE"=14, "TRIGGER SOURCE"=15, "TRIGGER ACTIVE"=16, "TRIGGER MODE"=17, "TRIGGER POLARITY"=18, "TRIGGER GLOBAL EXPOSURE"=19, "FIRST TRIGGER BEHAVIOR"=20, "TRIGGER TIMES"=21, "OUTPUT TRIGGER POLARITY"=22, "OUTPUT TRIGGER DELAY"=23, "OUTPUT TRIGGER PERIOD"=24, "TEMPERATURE"=25, "TEMPERATURE TARGET"=26, "SENSOR COOLER FAN"=27, "MECHANICAL SHUTTER"=28, "BACK FOCUS POSITION"=29, "FRAMEBUNDLE MODE"=30, "FRAMEBUNDLE NUMBER"=31, "LINEBUNDLE HEIGHT"=32, "TRIGGER CONNECTOR"=33, "IMAGE PIXEL TYPE"=34, "OUTPUT TRIGGER KIND"=35, "READOUT DIRECTION"=36, "CHANNEL SYNC"=37] ("Parameter")
        n226 = Dequeue Element(queue=w420) -> ()  [unwired: 2 in, 4 out]
        n227 = call "tm_stopcapture.vi"("error in (no error)"=w434, "Handle in"=w432) -> ("error out"=w433:errorcluster, "Handle out"=w431:u32)  [unwired: 8 in]
        n228 = call "tm_unpreparecapture.vi"("error in (no error)"=w433, "Handle in"=w431) -> ("error out"=w430:errorcluster, "Handle out"=w429:u32)  [unwired: 8 in]
        n229 = call "tm_setparameter.vi"("error in (no error)"=w430, "Value in"="t_exp", "Parameter"=w404, "Handle in"=w429) -> ("error out"=w406:errorcluster, "Handle out"=w405:u32)  [unwired: 6 in]
        n230 = call "tm_getparameter.vi"("error in (no error)"=w406, "Parameter"=w404, "Handle in"=w405) -> ("error out"=w402:errorcluster, "Value out"=w401:dbl, "Handle out"=w403:u32)  [unwired: 6 in]
        n231 = local write "t_exp"(w401) -> ()
        n232 = call "tm_setparameter.vi"("error in (no error)"=w402, "Value in"="Value in", "Parameter"=w427, "Handle in"=w403) -> ("error out"=w410:errorcluster, "Handle out"=w411:u32)  [unwired: 6 in]
        n233 = call "tm_preparecapture.vi"("error in (no error)"=w410, "Frames"=1, "Capture mode"=w426, "Handle in"=w411) -> ("error out"=w423:errorcluster, "Buffer Info"=w422:T4, "Handle out"=w424:u32)  [unwired: 4 in, 1 out]
        n234 = call "tm_startcapture_b.vi"("error in (no error)"=w423, "Handle in"=w424) -> ("error out"=w408:errorcluster, "Handle out"=w409:u32)  [unwired: 8 in]
        n235 = Unbundle(w422) -> ("height"=w418:u32, "width"=w419:u32)  [unwired: 1 out]
        n236 = property on="live" class="IntGraph (strict)"("XScale.Minimum"=0.0 ("X Scale.Range:Minimum"), "XScale.Maximum"=w418, "YScale.Minimum"=0.0 ("Y Scale.Range:Minimum"), "YScale.Maximum"=w419) -> ()  [unwired: 2 in, 2 out]
        n237 = Initialize Array(u16 0 ("element"), w418, w419) -> (w421:u16[][])
      }
      frame "close" {
        n238 = Release Queue(queue=w442) -> ()  [unwired: 2 in, 3 out]
      }
    }
  }
  n239 = while {
    tunnel: w25 -> [w451]
    shift-right: [w449] -> _
    shift-left: _ -> [w448]
    shift-right: [w446] -> _
    shift-left: -1 -> [w447]
    shift-right: [w445] -> _
    shift-left: _ -> [w444]
    tunnel: w23 -> [w443]
    stop <- w450 stop-if-true
    # "ISEG"
    n240 = Preview Queue Element(queue=w451, timeout in ms (-1)=w447) -> (element=w455:string)  [unwired: 1 in, 3 out]
    n241 = Match Pattern(string=w455, regular expression=":") -> (before substring=w453:string, after substring=w452:string)  [unwired: 1 in, 2 out]
    n242 = case shown="\"set\"" w453 {
      tunnel: w452 -> [_ w469 _ _ _]
      tunnel: w451 -> [_ w481 w523 w527 w531]
      tunnel: [_ _ _ _ TRUE] -> w450
      tunnel: [w458 w475 w521 w526 w528] -> w449
      tunnel: w448 -> [w460 w479 _ _ w528]
      tunnel: [0 _ _ _ _] -> w446
      tunnel: [w459 w476 T5 {"VISA Resource Name"="", "FP Notation"=FALSE, "Maximum Voltage"=0, "Maximum Current"=0} ("VISA Session Out") w524 w529] -> w445
      tunnel: w444 -> [w461 w480 w522 _ w529]
      tunnel: w443 -> [_ w464 _ _ _]
      frame "idle", Default {
        n243 = local read "Channel (A)"() -> (w462:enum16{"A", "B"})
        n244 = call "iseg NHQ xxx GetActualVoltage.vi"("error in (no error)"=w460, "Channel (A)"=w462, "VISA Session"=w461) -> ("error out"=w458:errorcluster, "Voltage"=w456:dbl, "VISA Session Out"=w459:T5)  [unwired: 5 in, 1 out]
        n245 = node(w456) -> (→"Actual Voltage":dbl[unit])
      }
      frame "set" {
        n246 = local read "Channel (A)"() -> (w472:enum16{"A", "B"})
        n247 = Dequeue Element(queue=w481) -> ()  [unwired: 2 in, 4 out]
        n248 = Match Pattern(string=w469, regular expression=":") -> (before substring=w468:string, after substring=w467:string)  [unwired: 1 in, 2 out]
        n249 = Fract/Exp String To Number(string=w468) -> (number=w471:dbl)  [unwired: 3 in, 1 out]
        n250 = call "iseg NHQ xxx SetNominalVoltage.vi"("error in (no error)"=w479, "Voltage (0 V)"=w471, "Channel (A)"=w472, "VISA Session"=w480) -> ("error out"=w482:errorcluster, "VISA Session Out"=w483:T5)  [unwired: 6 in]
        n251 = Equal?(x=w467, y="wait") -> (x = y?=w465:bool)
        n252 = call "iseg NHQ xxx StartVoltageChange.vi"("error in (no error)"=w482, "Channel (A)"=w472, "VISA Session"=w483) -> ("error out"=w477:errorcluster, "VISA Session Out"=w478:T5)  [unwired: 6 in, 1 out]
        n253 = case shown="True" w465 {
          tunnel: [w485 w495] -> w476
          tunnel: [w484 w487] -> w475
          tunnel: w478 -> [w485 w494]
          tunnel: w477 -> [w484 w493]
          tunnel: w471 -> [_ w492]
          tunnel: "volt_threshold" -> [_ w491]
          tunnel: "volt_timeout" -> [_ w490]
          tunnel: w472 -> [_ w489]
          tunnel: w464 -> [_ w488]
          frame False {
          }
          frame True {
            n254 = Tick Count (ms)() -> (millisecond timer value=w496:u32)
            n255 = while {
              shift-right: [w517] -> w495
              shift-left: w494 -> [w519]
              shift-right: [w504] -> w487
              shift-left: w493 -> [w518]
              tunnel: w489 -> [w516]
              tunnel: w491 -> [w513]
              tunnel: w496 -> [w511]
              tunnel: w490 -> [w509]
              tunnel: w492 -> [w508]
              tunnel: [w499] -> w486
              stop <- w505 stop-if-true
              n256 = Tick Count (ms)() -> (millisecond timer value=w512:u32)
              n257 = call "iseg NHQ xxx GetActualVoltage.vi"("error in (no error)"=w518, "Channel (A)"=w516, "VISA Session"=w519) -> ("error out"=w504:errorcluster, "Voltage"=w497:dbl, "VISA Session Out"=w517:T5)  [unwired: 5 in, 1 out]
              n258 = Absolute Value(x=w497) -> (abs(x)=w507:dbl)
              n259 = node(w497) -> (w498:dbl[unit])
              n260 = Subtract(x=w512, y=w511) -> (x-y=w510:u32)
              n261 = Subtract(x=w507, y=w508) -> (x-y=w515:dbl)
              n262 = local write "Actual Voltage"(w498) -> ()
              n263 = Absolute Value(x=w515) -> (abs(x)=w514:dbl)
              n264 = Greater?(x=w510, y=w509) -> (0:w503:bool)
              n265 = Less?(x=w514, y=w513) -> (x < y?=w506:bool)
              n266 = Or(x=w504, y=w503) -> (x .or. y?=w502:bool)
              n267 = Compound Arithmetic op=OR(w504, w506, w503) -> (w505:bool)
              n268 = Select(t="fail" ("element"), s=w502, f="done" ("element")) -> (s? t:f=w499:string)
            }
            n269 = Enqueue Element(queue=w488, element=w486) -> ()  [unwired: 2 in, 3 out]
          }
        }
      }
      frame "release" {
        n270 = Dequeue Element(queue=w523) -> ()  [unwired: 2 in, 4 out]
        n271 = call "iseg NHQ xxx Close.vi"("VISA session"=w522) -> ("error out"=w521:errorcluster)  [unwired: 14 in]
      }
      frame "init" {
        n272 = Dequeue Element(queue=w527) -> ()  [unwired: 2 in, 4 out]
        n273 = call "iseg NHQ xxx Initialize.vi"("VISA resource name"="VISA ISEG") -> ("VISA Session Out"=w524:T5, "error out"=w526:errorcluster)  [unwired: 13 in]
      }
      frame "close" {
        n274 = Release Queue(queue=w531) -> ()  [unwired: 2 in, 3 out]
      }
    }
    "error out" <- w449
  }
  n275 = while {
    shift-right: [w534] -> _
    shift-left: _ -> [w542]
    shift-right: [w540] -> _
    shift-left: 200 -> [w541]
    shift-right: [w538] -> _
    shift-left: _ -> [w537]
    tunnel: w20 -> [w535]
    tunnel: w17 -> [w532]
    stop <- w543 stop-if-true
    # "ESP301"
    n276 = Preview Queue Element(queue=w532, timeout in ms (-1)=w541) -> (queue out=w539:refnum<queue>, element=w547:string)  [unwired: 1 in, 2 out]
    n277 = Match Pattern(string=w547, regular expression=":") -> (before substring=w545:string, after substring=w544:string)  [unwired: 1 in, 2 out]
    n278 = case shown="\"idle\", Default" w545 {
      tunnel: w544 -> [_ w573 w613 _ _ _]
      tunnel: [_ _ _ _ _ TRUE] -> w543
      tunnel: [w557 w568 w609 w616 w624 w629] -> w534
      tunnel: w542 -> [w560 w577 w611 w618 _ w629]
      tunnel: w539 -> [_ w564 w605 w615 w625 w627]
      tunnel: [w558 w561 w610 refnum<visa-resource-name> refnum ("VISA resource name out") w623 w628] -> w538
      tunnel: w537 -> [w559 w576 w612 w619 _ w628]
      tunnel: "esp_axis" -> [w556 w562 w608 _ _ _]
      tunnel: w535 -> [_ w566 _ _ _ _]
      tunnel: [200 0 0 0 0 0] -> w533
      frame "idle", Default {
        n279 = call "Read Actual Position.vi"("error in (no error)"=w560, "Axis (1)"=w556, "VISA resource name"=w559) -> ("error out"=w557:errorcluster, "Position (units)"=w551:dbl, "VISA resource name out"=w558:refnum<visa-resource-name>)  [unwired: 2 in]
        "[mm]" <- w551
        n280 = local read "t0 @"() -> (w554:dbl)
        n281 = call "mm2time.vi"("fs?"=TRUE, "Offset (mm)"=w554, "distance (mm)"=w551) -> ("time in fs/ps seconds"=w552:dbl)
        n282 = Negate(x=w552) -> (-x=→"esp_pos_fs":dbl)
      }
      frame "abs" {
        n283 = Dequeue Element(queue=w564) -> ()  [unwired: 2 in, 4 out]
        n284 = Match Pattern(string=w573, regular expression=":") -> (before substring=w572:string, after substring=w571:string)  [unwired: 1 in, 2 out]
        n285 = Equal?(x=w571, y="confirm") -> (x = y?=w567:bool)
        n286 = Fract/Exp String To Number(string=w572) -> (number=w575:dbl)  [unwired: 3 in, 1 out]
        n287 = call "Move Absolute.vi"("error in (no error)"=w577, "Position (0 units)"=w575, "Axis (1)"=w562, "VISA resource name"=w576) -> ("error out"=w569:errorcluster, "VISA resource name out"=w563:refnum<visa-resource-name>)  [unwired: 2 in]
        n288 = case shown="True" w567 {
          tunnel: w569 -> [w579 w584]
          tunnel: [w579 w587] -> w568
          tunnel: w566 -> [_ w586]
          tunnel: w563 -> [w578 w582]
          tunnel: w562 -> [_ w581]
          tunnel: [w578 w580] -> w561
          frame False {
          }
          frame True {
            n289 = while {
              tunnel: w582 -> [w592]
              tunnel: w581 -> [w588]
              shift-right: [w596] -> w583
              shift-left: w584 -> [w591]
              tunnel: [w595] -> w580
              stop <- w598 continue-if-true
              n290 = call "Read Actual Position.vi"("error in (no error)"=w591, "Axis (1)"=w588, "VISA resource name"=w592) -> ("error out"=w589:errorcluster, "Position (units)"=w593:dbl, "VISA resource name out"=w590:refnum<visa-resource-name>)  [unwired: 2 in]
              n291 = local write "[mm]"(w593) -> ()
              n292 = Decrement(x=w588) -> (x-1=w594:i32)
              n293 = call "Get Controller Status.vi"("error in (no error)"=w589, "VISA resource name"=w590) -> ("error out"=w596:errorcluster, "Controller Status"=w604:T6, "VISA resource name out"=w595:refnum<visa-resource-name>)  [unwired: 2 in, 1 out]
              n294 = Unbundle(w604) -> ("Axis1 moving"=w603:bool, "Axis2 moving"=w602:bool, "Axis3 moving"=w601:bool, "Axis4 moving"=w600:bool)  [unwired: 12 out]
              n295 = Build Array(w603, w602, w601, w600) -> (w599:bool[])
              n296 = Index Array(array=w599, index=w594) -> (element=w597:bool)
              n297 = Or(x=w597, y=w596) -> (x .or. y?=w598:bool)
            }
            n298 = Send Notification(notification=TRUE, notifier=w586, error in (no error)=w583) -> (error out=w587:errorcluster)  [unwired: 1 out]
          }
        }
      }
      frame "rel" {
        n299 = Dequeue Element(queue=w605) -> ()  [unwired: 2 in, 4 out]
        n300 = Fract/Exp String To Number(string=w613) -> (number=w607:dbl)  [unwired: 3 in, 1 out]
        n301 = call "Move Relative.vi"("error in (no error)"=w611, "Position (0 units)"=w607, "Axis (1)"=w608, "VISA resource name"=w612) -> ("error out"=w609:errorcluster, "VISA resource name out"=w610:refnum<visa-resource-name>)  [unwired: 2 in]
      }
      frame "release" {
        n302 = Dequeue Element(queue=w615) -> ()  [unwired: 2 in, 4 out]
        n303 = call "Close.vi"("error in (no error)"=w618, "VISA resource name"=w619) -> ("error out"=w616:errorcluster)  [unwired: 9 in]
      }
      frame "init" {
        n304 = Dequeue Element(queue=w625) -> ()  [unwired: 2 in, 4 out]
        n305 = call "Initialize.vi"("VISA resource name"="esp_visa", "Serial Link (RS232)"=enum16{"RS232", "USB"}."RS232") -> ("VISA resource name out"=w623:refnum<visa-resource-name>, "error out"=w624:errorcluster)  [unwired: 7 in]
      }
      frame "close" {
        n306 = Release Queue(queue=w627) -> ()  [unwired: 2 in, 3 out]
      }
    }
    "esp301" <- w534
    n307 = case shown="No Error" w534 {
      tunnel: [w548 -1] -> w540
      tunnel: w533 -> [w548 _]
      frame No Error {
      }
      frame Error {
      }
    }
  }
  n308 = while {
    tunnel: w23 -> [w639]
    tunnel: w31 -> [w638]
    tunnel: w30 -> [w636]
    tunnel: w25 -> [w635]
    tunnel: w6 -> [w634]
    tunnel: w20 -> [w633]
    tunnel: w17 -> [w632]
    tunnel: w1 -> [w631]
    stop <- w637 stop-if-true
    # "coherent"
    n309 = Preview Queue Element(queue=w639) -> (element=w643:string)  [unwired: 2 in, 3 out]
    n310 = Match Pattern(string=w643, regular expression=":") -> (before substring=w641:string, after substring=w640:string)  [unwired: 1 in, 2 out]
    n311 = case shown="\"delay\"" w641 {
      tunnel: w640 -> [_ _ _ _ _]
      tunnel: w639 -> [w645 w649 w664 w748 _]
      tunnel: w638 -> [w646 _ w656 w746 _]
      tunnel: [TRUE _ _ _ _] -> w637
      tunnel: w636 -> [_ w648 w657 w745 _]
      tunnel: w635 -> [_ _ w658 _ _]
      tunnel: w634 -> [_ _ w659 _ _]
      tunnel: w633 -> [_ _ _ w762 _]
      tunnel: w632 -> [_ _ _ w743 _]
      tunnel: w631 -> [_ _ _ _ _]
      frame "close" {
        n312 = Release Queue(queue=w645) -> ()  [unwired: 2 in, 3 out]
        n313 = Release Queue(queue=w646) -> ()  [unwired: 2 in, 3 out]
      }
      frame "single" {
        n314 = Dequeue Element(queue=w649) -> ()  [unwired: 2 in, 4 out]
        n315 = Enqueue Element(queue=w648, element="snap") -> ()  [unwired: 2 in, 3 out]
      }
      frame "volt" {
        n316 = Flush Queue(queue=w664) -> (queue out=w660:refnum<queue>)  [unwired: 1 in, 2 out]
        n317 = local read "Path"() -> (w663:path)
        n318 = Build Path(base path=w663, name or relative path="head") -> (appended path=w651:path)
        n319 = Build Path(base path=w651, name or relative path="raw") -> (appended path=w653:path)
        n320 = Build Path(base path=w651, name or relative path="LUT.txt") -> (appended path=w654:path)
        n321 = Create Folder(path (use dialog)=w653) -> (created path=w652:path)  [unwired: 2 in, 2 out]
        n322 = while {
          tunnel: w660 -> [w665]
          tunnel: w659 -> [w688]
          tunnel: w658 -> [w682]
          tunnel: w657 -> [w681]
          tunnel: w656 -> [w680]
          tunnel: w654 -> [w675]
          tunnel: w652 -> [w674]
          shift-right: [w667] -> _
          shift-left: _ -> [w672]
          tunnel: [w665] -> w650
          i -> [w679]
          stop <- w666 stop-if-true
          n323 = call-poly <vilib>:"Ramp Pattern.vi"("start"="volt_start", "end"="volt_end", "samples"="volt_samples") -> ("Ramp Pattern"=w678:dbl[])  [unwired: 7 in, 1 out]
          n324 = Array Size(array=w678) -> (size(s)=w677:i32)
          n325 = Number To Fractional String(number=w678) -> (F-format string=w684:string[])  [unwired: 3 in]
          n326 = Multiply(x=w677, y=w679) -> (x*y=w676:i32)
          n327 = for {
            N -> [w691]
            tunnel: w688 -> [w718]
            tunnel: w665 -> [w725]
            tunnel: w684 -> [w708] mode=indexing
            tunnel: "set:" ("element") -> [w722]
            tunnel: w682 -> [w721]
            tunnel: w665 -> [w719]
            tunnel: w681 -> [w716]
            tunnel: w680 -> [w713]
            shift-right: [w693] -> w673
            shift-left: w672 -> [w711]
            tunnel: w676 -> [w710]
            tunnel: w675 -> [w707]
            tunnel: w674 -> [w706]
            tunnel: ":wait" ("element") -> [w692]
            i -> [w690]
            n328 = Concatenate Strings(w722, w708, w692) -> (w723:string)
            n329 = Add(x=w710, y=w690) -> (x+y=w709:i32)
            n330 = Divide(x=w690, y=w691) -> (x/y=→"Slide 2":dbl)
            n331 = Number To Decimal String(number=w709) -> (decimal integer string=w705:string)  [unwired: 1 in]
            n332 = Enqueue Element(queue=w721, element=w723, error in (no error)=w711) -> (error out=w720:errorcluster)  [unwired: 1 in, 2 out]
            n333 = Dequeue Element(queue=w719, error in (no error)=w720) -> (element=w702:string, error out=w700:errorcluster)  [unwired: 1 in, 2 out]
            n334 = Equal?(x="stop" ("y"), y=w702) -> (x = y?=w699:bool)
            n335 = call "inject_error.vi"("error in"=w700, "s"=w699) -> ("error out"=w701:errorcluster)  [unwired: 9 in]
            n336 = Enqueue Element(queue=w718, element="start", error in (no error)=w701) -> (error out=w715:errorcluster)  [unwired: 1 in, 2 out]
            n337 = Enqueue Element(queue=w716, element="snap", error in (no error)=w715) -> (error out=w714:errorcluster)  [unwired: 1 in, 2 out]
            n338 = Dequeue Element(queue=w713, error in (no error)=w714) -> (element=w704:dbl[][], error out=w712:errorcluster)  [unwired: 1 in, 2 out]
            n339 = Enqueue Element(queue=w718, element="ok", error in (no error)=w712) -> (error out=w724:errorcluster)  [unwired: 1 in, 2 out]
            n340 = Dequeue Element(queue=w725, error in (no error)=w724) -> (element=w696:string, error out=w695:errorcluster)  [unwired: 1 in, 2 out]
            n341 = Equal?(x="stop" ("y"), y=w696) -> (x = y?=w698:bool)
            n342 = call "inject_error.vi"("error in"=w695, "s"=w698) -> ("error out"=w694:errorcluster)  [unwired: 9 in]
            n343 = case shown="No Error" w694 {
              selector: w694 -> [w731 w741]
              tunnel: w708 -> [w730 _]
              tunnel: w707 -> [w737 _]
              tunnel: w706 -> [w736 _]
              tunnel: w705 -> [w735 _]
              tunnel: w704 -> [w733 _]
              tunnel: w696 -> [w732 _]
              tunnel: [w731 w741] -> w693
              frame No Error {
                n344 = Build Path(base path=w736, name or relative path=w735) -> (appended path=w734:path)
                n345 = Match Pattern(string=w732, regular expression=";") -> (before substring=w738:string, after substring=w729:string)  [unwired: 1 in, 2 out]
                n346 = Write to Binary File(file (use dialog)=w734, data=w733) -> ()  [unwired: 4 in, 3 out]
                n347 = Build Array(w735, w738, w729, w730) -> (w728:string[])
                n348 = call-poly <vilib>:"Write Delimited Spreadsheet.vi"("file path (dialog if empty)"=w737, "1D data"=w728, "append to file? (new file:F)"=TRUE) -> ()  [unwired: 11 in, 2 out]
              }
              frame Error {
              }
            }
          }
          n349 = Dequeue Element(queue=w665, error in (no error)=w673) -> (element=w670:string, error out=w667:errorcluster)  [unwired: 1 in, 2 out]
          n350 = Equal?(x="stop" ("y"), y=w670) -> (x = y?=w668:bool)
          n351 = Or(x=w668, y=w667) -> (x .or. y?=w666:bool)
        }
        n352 = Flush Queue(queue=w650) -> ()  [unwired: 1 in, 3 out]
      }
      frame "delay" {
        n353 = local read "Path"() -> (w761:path)
        n354 = Dequeue Element(queue=w748) -> ()  [unwired: 2 in, 4 out]
        n355 = Build Path(base path=w761, name or relative path="delayscan_header") -> (appended path=w750:path)
        n356 = call <vilib>:"Check if File or Folder Exists.vi"("path"=w750) -> ("file or folder exists?"=w752:bool, "dup path"=w751:path)  [unwired: 8 in, 1 out]
        n357 = case shown="False" w752 {
          tunnel: [w876 w877] -> w749
          tunnel: w751 -> [w875 w877]
          frame False {
            n358 = Create Folder(path (use dialog)=w875) -> (created path=w876:path)  [unwired: 2 in, 2 out]
          }
          frame True {
          }
        }
        n359 = call "create scan vectr.vi"("Table Control"="waypoints") -> ("Array"=w753:dbl[])
        n360 = Flush Queue(queue=w746) -> (queue out=w747:refnum<queue>)  [unwired: 1 in, 2 out]
        n361 = Array Size(array=w753) -> (size(s)=w756:i32)
        n362 = Build Path(base path=w749, name or relative path="times.txt") -> (appended path=w758:path)
        n363 = Flush Queue(queue=w743) -> (queue out=w742:refnum<queue>)  [unwired: 1 in, 2 out]
        n364 = Flush Queue(queue=w745) -> (queue out=w744:refnum<queue>)  [unwired: 1 in, 2 out]
        n365 = Initialize Array(0.0 ("element"), w756) -> (w754:dbl[])
        n366 = call-poly <vilib>:"Write Delimited Spreadsheet.vi"("file path (dialog if empty)"=w758, "1D data"=w753, "transpose? (no:F)"=TRUE) -> ()  [unwired: 11 in, 2 out]
        n367 = while {
          tunnel: w753 -> [w774]
          tunnel: w742 -> [w778]
          tunnel: w762 -> [w777]
          tunnel: w747 -> [w776]
          tunnel: w744 -> [w775]
          tunnel: w749 -> [w773]
          shift-right: [w771] -> _
          shift-left: w754 -> [w772]
          tunnel: w749 -> [w770]
          i -> [w767]
          stop <- w764 stop-if-true
          n368 = for {
            tunnel: w774 -> [w789] mode=indexing
            tunnel: w778 -> [w863]
            tunnel: w777 -> [w861]
            tunnel: w776 -> [w859]
            tunnel: w775 -> [w857]
            tunnel: w774 -> [w827]
            tunnel: w773 -> [w855]
            tunnel: w767 -> [w787]
            shift-right: [w825] -> w771
            shift-left: w772 -> [w828]
            tunnel: w770 -> [w823]
            tunnel: ["delayscan_stop"] -> w766
            i -> [w793]
            stop <- "delayscan_stop" stop-if-true
            w818 = T2 7 items=["Grayscale (U8)", "Grayscale (I16)", "Grayscale (SGL)", "Complex (CSG)", "RGB (U32)", "HSL (U32)", "RGB (U64)", "Grayscale (U16)"] ("Image Type")
            n369 = local read "t0 @"() -> (w868:dbl)
            n370 = Get Date/Time In Seconds() -> (seconds since 1Jan1904=w783:timestamp)
            n371 = Divide(x=w787, y=10000) -> (x/y=w853:dbl)
            n372 = Negate(x=w789) -> (-x=w790:dbl)
            n373 = Format Date/Time String(time format string (%c)="DelayScan_%Y%m%d_%H%M%S_", seconds (now)=w783) -> (date/time string=w779:string)  [unwired: 1 in]
            n374 = Divide(x=w793, y=10000) -> (x/y=w792:dbl)
            n375 = Number To Fractional String(number=w853) -> (F-format string=w852:string)  [unwired: 3 in]
            n376 = call "time2mm.vi"("fs[1]/ps[0]"=TRUE, "Offset (mm)"=w868, "time"=w790) -> ("position (mm)"=w786:dbl)
            n377 = Number To Fractional String(number=w792) -> (F-format string=w848:string)  [unwired: 3 in]
            n378 = Number To Fractional String(number=w786) -> (F-format string=w866:string)  [unwired: 3 in]
            n379 = String Subset(string=w852, offset (0)=2, length (rest)=4 ("length (rest)")) -> (substring=w850:string)
            n380 = String Subset(string=w848, offset (0)=2, length (rest)=4 ("length (rest)")) -> (substring=w781:string)
            n381 = Concatenate Strings("abs:" ("string"), w866, ":confirm" ("string")) -> (w864:string)
            n382 = Build Path(base path=w855, name or relative path=w850) -> (appended path=w796:path)
            n383 = call <vilib>:"Check if File or Folder Exists.vi"("path"=w796) -> ("file or folder exists?"=w797:bool, "dup path"=w798:path)  [unwired: 8 in, 1 out]
            n384 = Concatenate Strings(w779, w781) -> (w782:string)
            n385 = case shown="False" w797 {
              tunnel: [w871 w872] -> w795
              tunnel: w798 -> [w870 w872]
              frame False {
                n386 = Create Folder(path (use dialog)=w870) -> (created path=w871:path)  [unwired: 2 in, 2 out]
              }
              frame True {
              }
            }
            n387 = Enqueue Element(queue=w863, element=w864) -> (error out=w862:errorcluster)  [unwired: 2 in, 2 out]
            n388 = Concatenate Strings(w782, ".bin" ("string")) -> (w803:string)
            n389 = Concatenate Strings(w782, ".png" ("string")) -> (w801:string)
            n390 = Wait on Notification(notifier=w861, error in (no error)=w862) -> (error out=w860:errorcluster)  [unwired: 2 in, 3 out]
            n391 = Build Path(base path=w795, name or relative path=w803) -> (appended path=w824:path)
            n392 = Build Path(base path=w823, name or relative path="positions.txt") -> (appended path=w821:path)
            n393 = property on="live" class="IntGraph (strict)"() -> ("CrsrLis"=w847:T7)  [unwired: 2 in, 2 out]
            n394 = Build Path(base path=w795, name or relative path=w801) -> (appended path=w800:path)
            n395 = Enqueue Element(queue=w857, element="snap", error in (no error)=w860) -> (error out=w858:errorcluster)  [unwired: 1 in, 2 out]
            n396 = Index Array(array=w847) -> (element #1=w846:T8, element #2=w845:T8)  [unwired: 2 in]
            n397 = Unbundle By Name(w846) -> ("Position.X"=w844:dbl, "Position.Y"=w842:dbl)
            n398 = Unbundle By Name(w845) -> ("Position.X"=w843:dbl, "Position.Y"=w841:dbl)
            n399 = Dequeue Element(queue=w859, error in (no error)=w858) -> (element=w799:dbl[][])  [unwired: 1 in, 3 out]
            n400 = Build Array(w844, w843) -> (w840:dbl[])
            n401 = Build Array(w842, w841) -> (w839:dbl[])
            n402 = Array Max & Min(array=w840) -> (max value=w838:dbl, min value=w836:dbl)  [unwired: 2 out]
            n403 = Array Max & Min(array=w839) -> (max value=w837:dbl, min value=w834:dbl)  [unwired: 2 out]
            n404 = Write to Binary File(file (use dialog)=w824, data=w799) -> ()  [unwired: 4 in, 3 out]
            n405 = Subtract(x=w836, y=w838) -> (x-y=w835:dbl)
            n406 = Subtract(x=w834, y=w837) -> (x-y=w833:dbl)
            n407 = Array Subset(array=w799, index (row)=w836, length (row)=w835, index (col)=w834, length (col)=w833) -> (w832:dbl[][])
            n408 = Array Size(array=w799) -> (size(s)=w830:i32[])
            n409 = Add Array Elements(numeric array=w832) -> (sum=w831:dbl)
            n410 = Multiply Array Elements(1:w830) -> (0:w829:i32)
            n411 = Divide(x=w831, y=w829) -> ()  [unwired: 1 out]
            n412 = for {
              tunnel: w799 -> [w874] mode=indexing
              tunnel: [w873] -> w813 mode=indexing
              n413 = Reverse 1D Array(array=w874) -> (reversed array=w873:dbl[])
            }
            n414 = Replace Array Subset(array=w828, new element=w786, index=w793) -> (w825:dbl[])
            n415 = Bundle("Array"=w827, w825) -> (→"XY Graph":cluster{"Array":dbl[], dbl[]})  [unwired: 1 in]
            n416 = call-poly <vilib>:"Write Delimited Spreadsheet.vi"("file path (dialog if empty)"=w821, "format (%.3f)"="%.6f", "1D data"=w825, "transpose? (no:F)"=TRUE) -> ()  [unwired: 10 in, 2 out]
            n417 = Transpose 2D Array(2D array=w813) -> (transposed array=w807:dbl[][])
            n418 = Array Max & Min(array=w807) -> (min value=w806:dbl)  [unwired: 3 out]
            n419 = Subtract(x=w807, y=w806) -> (x-y=w805:dbl[][])
            n420 = call "IMAQ Create"("Image Name"="untitled", "Image Type"=w818) -> ("New Image"=w819:T3)  [unwired: 3 in, 1 out]
            n421 = Array Max & Min(array=w805) -> (max value=w812:dbl)  [unwired: 3 out]
            n422 = Divide(x=w805, y=w812) -> (x/y=w811:dbl[][])
            n423 = Multiply(x=w811, y=255) -> (x*y=w809:dbl[][])
            n424 = To Unsigned Word Integer(number=w809) -> (unsigned 16bit integer=w808:u16[][])
            n425 = call "IMAQ ArrayToImage"("Image Pixels (U16)"=w808, "Image"=w819) -> ("Image Out"=w817:T3)  [unwired: 8 in, 1 out]
            n426 = call-poly "IMAQ Write File 2"("Image Quality"=u32 1000, "File Path"=w800, "Image"=w817) -> ("Image Out (duplicate)"=w815:T3)  [unwired: 7 in, 1 out]
            n427 = call "IMAQ Dispose"("Image"=w815) -> ()  [unwired: 5 in, 1 out]
          }
          n428 = Increment(x=w767) -> (x+1=w768:i32)
          n429 = Greater Or Equal?(x=w768, y="iterations") -> (x >= y?=w765:bool)
          n430 = Or(x=w766, y=w765) -> (x .or. y?=w764:bool)
        }
      }
      frame "idle", Default {
      }
    }
  }
